vi "main 0.9.4.testing.vi"() -> ()   [LabVIEW 2020]
uses:
  subvi/Newport ESP301/Newport ESP301.lvlib
  subvi/sp_manip.llb/sp_manip_lib.lvlib
  subvi/sp_manip.llb/tcp_gateway.lvlib
  subvi/PHOIBOS/DEFINITIONS/DEF_dev_type.ctl
  subvi/PHOIBOS/DEFINITIONS/DEF_dev_state.ctl
  <vilib>/Utility/file.llb/Write Delimited Spreadsheet (DBL).vi
  <vilib>/Utility/file.llb/Read Delimited Spreadsheet (string).vi
  <vilib>/Analysis/NI_AALBase.lvlib
  <vilib>/Analysis/1siggen.llb/Ramp Pattern by Samples.vi
  <vilib>/DAQmx/create/channels.llb/DAQmx Create Channel (AI-Voltage-Basic).vi
  <vilib>/DAQmx/read.llb/DAQmx Read (Analog DBL 1Chan 1Samp).vi
panel:
  out "Pics L":i32
  out "Pics NL":i32
  out "Voltage":dbl format="%0.2f"
  out "sideimg 2":dbl[][](graph)
  in  "Frame trigger \n(High Performance and QE only)":u16
  in  "Operating mode\nHP & QE / HS & DiCam Pro":u32
  out "Waveform Chart":dbl(graph)
  out "G2 X":cluster{dbl[], "Ramp Pattern":dbl[]}(graph)={array[344 elements], "Ramp Pattern"=[5593.0, 5541.0, 5578.0, 5573.0, 5542.0, 5582.0, 5523.0, 5570.0, 5578.0, 5560.0, 5581.0, 5542.0, 5577.0, 5517.0, 5599.0, 5558.0, 5549.0, 5571.0, 5527.0, 5574.0, 5565.0, 5561.0, 5570.0, 5531.0, 5576.0, 5531.0, 5576.0, 5554.0, 5523.0, 5573.0, 5536.0, 5555.0, 5539.0, 5549.0, 5543.0, 5541.0, 5581.0, 5523.0, 5548.0, 5528.0, 5558.0, 5565.0, 5537.0, 5556.0, 5521.0, 5538.0, 5549.0, 5532.0, 5562.0, 5512.0, 5555.0, 5549.0, 5536.0, 5542.0, 5511.0, 5567.0, 5526.0, 5549.0, 5545.0, 5543.0, 5562.0, 5518.0, 5561.0, 5490.0, 5542.0, 5522.0, 5529.0, 5542.0, 5521.0, 5556.0, 5511.0, 5541.0, 5534.0, 5512.0, 5569.0, 5525.0, 5547.0, 5507.0, 5533.0, 5533.0, 5501.0, 5555.0, 5497.0, 5517.0, 5526.0, 5519.0, 5565.0, 5503.0, 5548.0, 5496.0, 5544.0, 5523.0, 5534.0, 5533.0, 5501.0, 5529.0, 5494.0, 5523.0, 5526.0, 5519.0, 5539.0, 5493.0, 5508.0, 5532.0, 5504.0, 5546.0, 5540.0, 5550.0, 5488.0, 5556.0, 5535.0, 5510.0, 5535.0, 5515.0, 5543.0, 5475.0, 5538.0, 5528.0, 5504.0, 5523.0, 5502.0, 5535.0, 5473.0, 5503.0, 5501.0, 5531.0, 5525.0, 5490.0, 5524.0, 5484.0, 5520.0, 5506.0, 5492.0, 5516.0, 5477.0, 5511.0, 5487.0, 5509.0, 5496.0, 5467.0, 5538.0, 5494.0, 5512.0, 5497.0, 5498.0, 5526.0, 5482.0, 5506.0, 5466.0, 5522.0, 5489.0, 5512.0, 5518.0, 5475.0, 5547.0, 5480.0, 5569.0, 5504.0, 5485.0, 5528.0, 5506.0, 5529.0, 5468.0, 5524.0, 5507.0, 5518.0, 5511.0, 5471.0, 5525.0, 5480.0, 5482.0, 5510.0, 5506.0, 5522.0, 5475.0, 5540.0, 5477.0, 5511.0, 5514.0, 5500.0, 5497.0, 5484.0, 5536.0, 5476.0, 5485.0, 5527.0, 5509.0, 5529.0, 5495.0, 5504.0, 5496.0, 5519.0, 5512.0, 5469.0, 5506.0, 5465.0, 5502.0, 5481.0, 5508.0, 5519.0, 5499.0, 5515.0, 5476.0, 5496.0, 5502.0, 5499.0, 5494.0, 5477.0, 5541.0, 5477.0, 5512.0, 5497.0, 5472.0, 5511.0, 5471.0, 5503.0, 5507.0, 5504.0, 5477.0, 5479.0, 5508.0, 5481.0, 5522.0, 5517.0, 5516.0, 5505.0, 5502.0, 5491.0, 5481.0, 5512.0, 5484.0, 5500.0, 5478.0, 5493.0, 5529.0, 5492.0, 5518.0, 5471.0, 5518.0, 5490.0, 5513.0, 5497.0, 5488.0, 5517.0, 5477.0, 5524.0, 5464.0, 5495.0, 5514.0, 5495.0, 5522.0, 5477.0, 5490.0, 5535.0, 5489.0, 5491.0, 5491.0, 5515.0, 5473.0, 5504.0, 5505.0, 5515.0, 5510.0, 5473.0, 5521.0, 5475.0, 5537.0, 5499.0, 5505.0, 5509.0, 5460.0, 5509.0, 5473.0, 5489.0, 5500.0, 5464.0, 5522.0, 5471.0, 5528.0, 5475.0, 5502.0, 5494.0, 5511.0, 5516.0, 5486.0, 5528.0, 5471.0, 5492.0, 5477.0, 5491.0, 5531.0, 5486.0, 5549.0, 5498.0, 5524.0, 5482.0, 5495.0, 5505.0, 5476.0, 5512.0, 5444.0, 5512.0, 5498.0, 5471.0, 5489.0, 5462.0, 5502.0, 5459.0, 5503.0, 5489.0, 5493.0, 5498.0, 5461.0, 5505.0, 5495.0, 5503.0, 5459.0, 5501.0, 5515.0, 5459.0, 5510.0, 5469.0, 5504.0, 5499.0, 5505.0, 5524.0, 5477.0, 5527.0, 5477.0, 5475.0, 5495.0, 5482.0, 5514.0, 5481.0, 5499.0, 5481.0, 5482.0, 5498.0, 5460.0, 5469.0, 5471.0, 5519.0, 5495.0, 5485.0]}
  in  "reset every n pics":bool
  in  "pics2avg":i32=50
  in  "abort acq.":bool
  out "G2 Y":cluster{dbl[], "Ramp Pattern":dbl[]}(graph)={[5738.0, 5692.0, 5562.0, 5630.0, 5633.0, 5616.0, 5523.0, 5622.0, 5406.0, 5598.0, 5416.0, 5403.0, 5579.0, 5325.0, 5504.0, 5402.0, 5538.0, 5568.0, 5460.0, 5494.0, 5367.0, 5597.0, 5434.0, 5448.0, 5339.0, 5434.0, 5460.0, 5482.0, 5646.0, 5720.0, 5704.0, 5628.0, 5672.0, 5511.0, 5420.0, 5539.0, 5543.0, 5421.0, 5486.0, 5508.0, 5537.0, 5586.0, 5460.0, 5547.0, 5433.0, 5488.0, 5552.0, 5538.0, 5528.0, 5482.0, 5406.0, 5458.0, 5644.0, 5485.0, 5443.0, 5485.0, 5385.0, 5413.0, 5472.0, 5571.0, 5640.0, 5602.0, 5462.0, 5477.0, 5408.0, 5396.0, 5445.0, 5638.0, 5383.0, 5571.0, 5372.0, 5519.0, 5426.0, 5462.0, 5481.0, 5626.0, 5326.0, 5458.0, 5471.0, 5366.0, 5394.0, 5363.0, 5551.0, 5596.0, 5452.0, 5470.0, 5600.0, 5533.0, 5573.0, 5544.0, 5671.0, 5595.0, 5423.0, 5550.0, 5557.0, 5416.0, 5404.0, 5478.0, 5448.0, 5512.0, 5505.0, 5575.0, 5434.0, 5436.0, 5600.0, 5487.0, 5607.0, 5463.0, 5606.0, 5540.0, 5521.0, 5581.0, 5472.0, 5555.0, 5576.0, 5612.0, 5529.0, 5473.0, 5454.0, 5455.0, 5500.0, 5650.0, 5451.0, 5445.0, 5423.0, 5376.0, 5389.0, 5491.0, 5536.0, 5525.0, 5440.0, 5707.0, 5414.0, 5532.0, 5400.0, 5668.0, 5706.0, 5515.0, 5431.0, 5400.0, 5439.0, 5471.0, 5627.0, 5691.0, 5569.0, 5718.0, 5614.0, 5523.0, 5436.0, 5432.0, 5419.0, 5516.0, 5469.0, 5467.0, 5530.0, 5598.0, 5501.0, 5476.0, 5457.0, 5460.0, 5606.0, 5456.0, 5429.0, 5586.0, 5504.0, 5546.0, 5516.0, 5466.0, 5650.0, 5593.0, 5605.0, 5515.0, 5414.0, 5623.0, 5581.0, 5651.0, 5574.0, 5519.0, 5672.0, 5621.0, 5496.0, 5382.0, 5496.0, 5620.0, 5542.0, 5422.0, 5492.0, 5515.0, 5549.0, 5402.0, 5472.0, 5547.0, 5515.0, 5641.0, 5451.0, 5667.0, 5622.0, 5511.0, 5506.0, 5608.0, 5647.0, 5584.0, 5714.0, 5490.0, 5534.0, 5463.0, 5566.0, 5573.0, 5570.0, 5582.0, 5613.0, 5504.0, 5550.0, 5594.0, 5576.0, 5677.0, 5675.0, 5681.0, 5681.0, 5434.0, 5434.0, 5405.0, 5473.0, 5522.0, 5427.0, 5533.0, 5582.0, 5427.0, 5529.0, 5548.0, 5341.0, 5521.0, 5539.0, 5435.0, 5457.0, 5511.0, 5406.0, 5412.0, 5620.0, 5609.0, 5609.0, 5469.0, 5577.0, 5661.0, 5673.0, 5518.0, 5463.0, 5562.0, 5723.0, 5719.0, 5487.0, 5485.0, 5683.0, 5501.0, 5604.0, 5328.0], "Ramp Pattern"=[0.0, 1.003921568627451, 2.007843137254902, 3.011764705882353, 4.015686274509804, 5.019607843137255, 6.023529411764706, 7.027450980392157, 8.031372549019608, 9.035294117647059, 10.03921568627451, 11.04313725490196, 12.047058823529412, 13.050980392156863, 14.054901960784314, 15.058823529411764, 16.062745098039215, 17.066666666666666, 18.070588235294117, 19.07450980392157, 20.07843137254902, 21.08235294117647, 22.08627450980392, 23.090196078431372, 24.094117647058823, 25.098039215686274, 26.101960784313725, 27.105882352941176, 28.109803921568627, 29.113725490196078, 30.11764705882353, 31.12156862745098, 32.12549019607843, 33.129411764705885, 34.13333333333333, 35.13725490196079, 36.141176470588235, 37.14509803921569, 38.14901960784314, 39.15294117647059, 40.15686274509804, 41.16078431372549, 42.16470588235294, 43.168627450980395, 44.17254901960784, 45.1764705882353, 46.180392156862744, 47.1843137254902, 48.188235294117646, 49.1921568627451, 50.19607843137255, 51.2, 52.20392156862745, 53.207843137254905, 54.21176470588235, 55.21568627450981, 56.219607843137254, 57.22352941176471, 58.227450980392156, 59.23137254901961, 60.23529411764706, 61.23921568627451, 62.24313725490196, 63.247058823529414, 64.25098039215686, 65.25490196078431, 66.25882352941177, 67.26274509803922, 68.26666666666667, 69.27058823529411, 70.27450980392157, 71.27843137254902, 72.28235294117647, 73.28627450980392, 74.29019607843138, 75.29411764705883, 76.29803921568627, 77.30196078431372, 78.30588235294118, 79.30980392156863, 80.31372549019608, 81.31764705882352, 82.32156862745099, 83.32549019607843, 84.32941176470588, 85.33333333333333, 86.33725490196079, 87.34117647058824, 88.34509803921569, 89.34901960784313, 90.3529411764706, 91.35686274509804, 92.36078431372549, 93.36470588235294, 94.3686274509804, 95.37254901960785, 96.37647058823529, 97.38039215686274, 98.3843137254902, 99.38823529411765, 100.3921568627451, 101.39607843137254, 102.4, 103.40392156862745, 104.4078431372549, 105.41176470588235, 106.41568627450981, 107.41960784313726, 108.4235294117647, 109.42745098039215, 110.43137254901961, 111.43529411764706, 112.43921568627451, 113.44313725490196, 114.44705882352942, 115.45098039215686, 116.45490196078431, 117.45882352941176, 118.46274509803922, 119.46666666666667, 120.47058823529412, 121.47450980392156, 122.47843137254903, 123.48235294117647, 124.48627450980392, 125.49019607843137, 126.49411764705883, 127.49803921568628, 128.50196078431372, 129.50588235294117, 130.50980392156862, 131.51372549019607, 132.51764705882354, 133.521568627451, 134.52549019607844, 135.52941176470588, 136.53333333333333, 137.53725490196078, 138.54117647058823, 139.54509803921567, 140.54901960784315, 141.5529411764706, 142.55686274509804, 143.5607843137255, 144.56470588235294, 145.5686274509804, 146.57254901960783, 147.57647058823528, 148.58039215686276, 149.5843137254902, 150.58823529411765, 151.5921568627451, 152.59607843137255, 153.6, 154.60392156862744, 155.6078431372549, 156.61176470588236, 157.6156862745098, 158.61960784313726, 159.6235294117647, 160.62745098039215, 161.6313725490196, 162.63529411764705, 163.6392156862745, 164.64313725490197, 165.64705882352942, 166.65098039215687, 167.65490196078431, 168.65882352941176, 169.6627450980392, 170.66666666666666, 171.6705882352941, 172.67450980392158, 173.67843137254903, 174.68235294117648, 175.68627450980392, 176.69019607843137, 177.69411764705882, 178.69803921568626, 179.7019607843137, 180.7058823529412, 181.70980392156864, 182.71372549019608, 183.71764705882353, 184.72156862745098, 185.72549019607843, 186.72941176470587, 187.73333333333332, 188.7372549019608, 189.74117647058824, 190.7450980392157, 191.74901960784314, 192.75294117647059, 193.75686274509803, 194.76078431372548, 195.76470588235293, 196.7686274509804, 197.77254901960785, 198.7764705882353, 199.78039215686275, 200.7843137254902, 201.78823529411764, 202.7921568627451, 203.79607843137254, 204.8, 205.80392156862746, 206.8078431372549, 207.81176470588235, 208.8156862745098, 209.81960784313725, 210.8235294117647, 211.82745098039214, 212.83137254901962, 213.83529411764707, 214.8392156862745, 215.84313725490196, 216.8470588235294, 217.85098039215686, 218.8549019607843, 219.85882352941175, 220.86274509803923, 221.86666666666667, 222.87058823529412, 223.87450980392157, 224.87843137254902, 225.88235294117646, 226.8862745098039, 227.89019607843136, 228.89411764705883, 229.89803921568628, 230.90196078431373, 231.90588235294118, 232.90980392156862, 233.91372549019607, 234.91764705882352, 235.92156862745097, 236.92549019607844, 237.9294117647059, 238.93333333333334, 239.93725490196078, 240.94117647058823, 241.94509803921568, 242.94901960784313, 243.95294117647057, 244.95686274509805, 245.9607843137255, 246.96470588235294, 247.9686274509804, 248.97254901960784, 249.9764705882353, 250.98039215686273, 251.98431372549018, 252.98823529411766, 253.9921568627451, 254.99607843137255, 256.0]}
  out "ETA":timestamp=timestamp(3543843884.995538 s since 1904-01-01) format="%<%H:%M:%S>T"
  out "acq. imgs":i32=30
  out "snap_prog":dbl(slide)=1.0 scale=0.0..1.0
  in  "BasePath":path=path "Z:/PESdata"
  in  "cam_liveavg":bool caption="live average"
  out "cam_fps":dbl=20.079713544692744 caption="FPS" format="%.1g"
  out "sideimg":dbl[][](graph)
  in  "RunNumber":u16=77
  out "sum":dbl=4126991.0 format="%#.2g"
  out "max":dbl=54.0
  out "mainimg":dbl[][](graph)
  out "ESP_con?":bool=TRUE caption="ESP301"
  out "phoib_con?":bool caption="PHOIBOS"
  out "manip_con?":bool caption="manipulator"
  out "cam_con?":bool caption="camera"
  in  "main_close":bool
  in  "Tab Control":T1(tab)
  in  "manip_deltas":dbl[](array[numeric])=[0.0, 0.0, 0.0, 0.0, 10.0, 0.0] caption="delta" format="%#.5g"
  in  "aq.mode":enum32{"Radio Selection 1", "Radio Selection 2"}(radio)=enum."Radio Selection 2"
  in  "dark avg":i32=100
  in  "averages":i32=30 caption="N"
  in  "ESP_delta":dbl caption="relative [mm]"
  in  "ESP_-":bool
  in  "ESP_+":bool
  in  "ESP_go":bool
  in  "ESP_dest_t":dbl=250.17307139859977 caption="[fs]"
  in  "ESP_dest":dbl=31.304 caption="[mm]"
  in  "ESP_set_t0":bool
  in  "phoib_I_6s":dbl=3200.0
  in  "phoib_I_5s":dbl=1650.0
  in  "phoib_I_4s":dbl=4.558
  in  "phoib_I_3s":dbl=-7.0
  in  "phoib_I_2s":dbl=20.0
  in  "phoib_I_1s":dbl=22.0
  in  "phoib_standby":bool
  in  "phoib_set":bool
  out "phoib_I_6":dbl caption="Screen Voltage"
  out "phoib_I_5":dbl caption="Detctor Voltage"
  out "phoib_I_4":dbl caption="Work Function"
  out "phoib_I_3":dbl caption="Coil Current"
  out "phoib_I_2":dbl caption="Pass Energy"
  out "phoib_I_1":dbl caption="Kinetic Energy"
  out "Saved Positions":string[][](table)=[["ertwertwert", "-2.299945", "-2.030214", "38.900024", "50.000762", "0.000887", "-97.998082"], ["uztgugt", "-14.999451", "-13.638894", "442.380066", "13.998380", "-1.893758", "-76.305838"], ["asdf", "-14.999451", "-13.638894", "442.380066", "13.998380", "-1.893758", "-76.305838"], ["test3", "-14.999451", "-13.638894", "441.380066", "13.998380", "-1.893758", "-76.305838"]]
  in  "Save Pos":bool
  in  "Load":bool
  in  "Delete":bool
  in  "ManipRel +":bool
  in  "ManipRel -":bool
  in  "Move Abs":bool
  in  "stop manip":bool
  in  "dest":dbl[](array[numeric])=[-2.6172862113166087, -0.009888298846365134, 68.5008544921875, -46.36280498847848, 1.1073518432055398, -218.56360350415366] caption="destination" format="%#.5g"
  out "axis":string[](array[string])=["x", "y", "z", "polar", "tilt", "azimut"]
  out "pos":dbl[](array[numeric])=[-2.6172862113166087, -0.009888298846365134, 68.5008544921875, -46.363686276590336, 11.108982061941884, -218.56360350415366] caption="position" format="%.5f"
  in  "Mode":T2(ring)=enum."WideAngleMode"
  in  "VoltageRange":enum16{"3.5kV", "1.5kV", "400V", "100V", "10V"}(ring)=enum."400V"
  out "ESP_pos":dbl=31.4539 caption="Position"
  out "ESP_delay":dbl=1000.0251574040756 caption="Delay"
  out "ESP_t0":dbl=31.304 caption="Time Zero @"
  out "phoib_I_7":dbl caption="Conversion Voltage"
  in  "phoib_I_7s":dbl=-16.0
  in  "phoib_I_8s":dbl=0.0039
  in  "phoib_I_9s":dbl=0.0039
  out "phoib_I_8":dbl caption="FD1"
  out "phoib_I_9":dbl caption="FD2"
  in  "gain":bool
  in  "exposure [ms]":u32=1
  in  "binning":u16(ring)=2 items=["X 1", "X 2", "X 4", "X 8"]
  in  "cam_dark?":bool caption="subtract dark?"
  in  "cam_dark":bool
  in  "cam_saveimg":bool
  in  "e-size":u8
  in  "lower threshold":i32=-100
  in  "count?":bool
  in  "ROI Left":i32=1
  in  "ROI Right":i32=43
  in  "ROI Top":i32=1
  in  "ROI Bottom":i32=33
  out "moving?":bool[](array[boolean])
  in  "delscan_abort 2":bool
  in  "delscan_go 2":bool
  in  "delscan_finishIteration 2":bool
  out "del_ETA":timestamp=timestamp(3543843871.185777 s since 1904-01-01) format="%<%H:%M:%S>T"
  out "time / step":dbl=2.792118032773336
  out "duration [HH:MM:SS]":dbl=55.62603882380894 format="%<%H:%M:%S>t"
  out "disk [MB]":dbl=11.613000000000001
  out "RAM [MB]":dbl=2.765
  out "total steps":dbl=20.0
  out "delaypoints":dbl=5.0
  in  "generate delay table":bool
  in  "load delay table":bool
  in  "delay table [fs]":string[][](table)=[["-1000.000000"], ["-500.000000"], ["0.000000"], ["500.000000"], ["1000.000000"]]
  in  "delscan_iters":u32=4 caption="iterations"
  out "scangraph":cluster{"delaypoints":dbl[], dbl[]}(graph)={"delaypoints"=[-1000.0, -500.0, 0.0, 500.0, 1000.0], [56872639.0, 56944859.59999999, 56835838.7999999, 56879783.599999934, 56864774.39999998]}
  in  "delscan_abort":bool
  out "delscan_progress":u32(slide)=5 scale=0.0..5.0
  in  "delscan_go":bool
  out "delscan_pos":dbl=31.453896228999998 caption="stage pos [mm]"
  in  "delscan_end":dbl=1000.0 caption="end [fs]"
  in  "delscan_stepsize":dbl=500.0 caption="stepsize [fs]"
  in  "delscan_start":dbl=-1000.0 caption="start [fs]"
  out "iteration":i32=5
  in  "delscan_finishIteration":bool
  in  "manip_scan_steps":u32=3
  in  "Optimize":bool
  in  "manip_scan_delta":dbl[](array[numeric])=[0.0, 0.0, 0.0, 0.0, 1.0, 0.0] caption="delta" format="%#.5g"
  out "delscan_progress 2":u32(slide)=2 scale=0.0..3.0
  in  "abort":bool
  in  "dev_bench":bool
  out "x/y":dbl
  out "1/x":dbl
  in  "stop":bool
  out "voltage out":dbl
  in  "manip_init":bool
  in  "manip_release":bool
  in  "phoib_init":bool
  in  "phoib_release":bool
  in  "ESP_init":bool
  in  "ESP_release":bool
  in  "ESP301 VISA":refnum<visa-resource-name>="COM8"
  in  "board number":i32
  in  "cam_init":bool
  in  "cam_release":bool
  out "cam_error":errorcluster
  out "phoib_error":errorcluster
  out "state":T3 items=["Off"=-1, "Standby"=0, "On"=1]
  in  "ESP Axis":i32=1 min=1 max=3
  out "error out":errorcluster
  out "error out 2":errorcluster={"status"=TRUE, "code"=1, "source"="TCP Write in sp_manip_lib.lvlib:sp_manip_disconnect.vi->main 0.9.1.vi"}
  # "0 = sequential\n1 = simultaneous"
  # "0 = internal\n1 = external rising\n2 = external falling"
  # "camera"
  # "analyzer"
  # "manipulator"
  # "aquisition"
  # "delay stage"
  # "Position"
  # "Destination"
  # "X\nY\nZ\npolar\ntilt\nazimut"
  # "camera"
  # "phoibos"
  # "ESP301"
  # "manipulator"
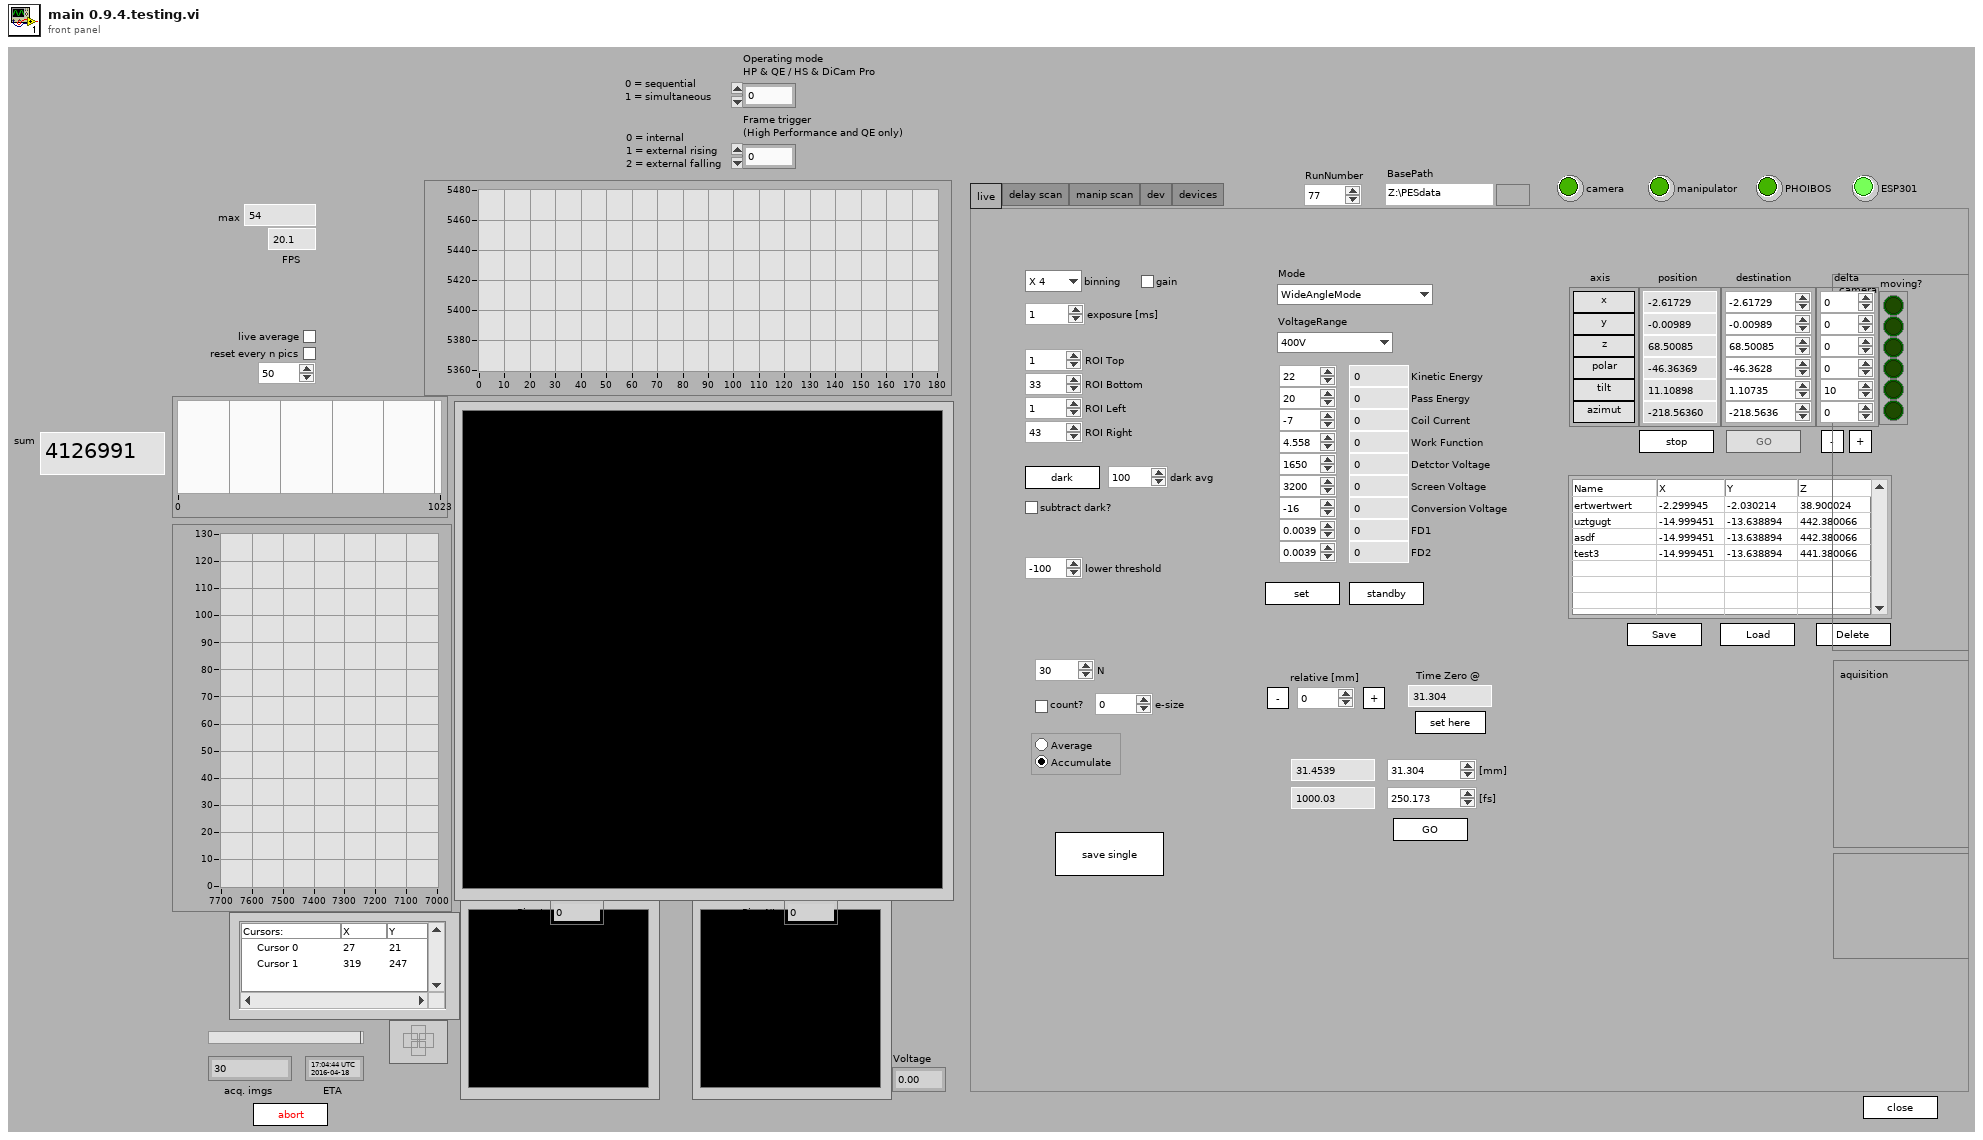
[diagram p1: front panel]
types:
  T1 = enum32{"live", "delay scan", "manip scan", "dev", "devices"}
  T2 = enum16{"HighMagnification", "MediumMagnification", "LowMagnification", "HighAngularDispersion", "MediumAngularDispersion", "LowAngularDispersion", "WideAngleMode", "LargeArea", "MediumArea", "SmallArea", "HighMagnification2", "SmallArea2", "ImagingMode"}
  T3 = typedef "DEF_dev_state.ctl" = i32
  T4 = typedef "LVCursorListTypeDef.ctl" = cluster{"Name":string, "Color":u32, "Style":u8, "Point Style":u8, "Name Visible":bool, "Allow Drag":bool, "Cursor Mode":u32, "Plot":i32, "Index":i32, "Position":cluster{"X":dbl, "Y":dbl}, "X Scale":u32, "Y Scale":u32, "Watch Plots":i32[], "Watch All Plots":bool, "Plot Area":i32, "Label Offset":cluster{"X":dbl, "Y":dbl}}[]
  T5 = cluster{"delay pointss [fs]":dbl[], "Intensity Chart":dbl[]}
  T6 = cluster{"Camera type":u32, "Operating mode\nHP & QE / HS & DiCam Pro ":u32, "Frame trigger \n(High Performance and QE only)":u16, "Sequence trigger":u16, "Low Light\n(QE only)":bool, "Gain":bool, "Horzontal\nbinning":u16, "Vertical\nbinning ":u16, "ROI Left":i32, "ROI Right":i32, "ROI Top":i32, "ROI Bottom":i32}
  T7 = cluster{"Name":string, "Color":u32, "Style":u8, "Point Style":u8, "Name Visible":bool, "Allow Drag":bool, "Cursor Mode":u32, "Plot":i32, "Index":i32, "Position":cluster{"X":dbl, "Y":dbl}, "X Scale":u32, "Y Scale":u32, "Watch Plots":i32[], "Watch All Plots":bool, "Plot Area":i32, "Label Offset":cluster{"X":dbl, "Y":dbl}}
  T8 = cluster{"Axis_Name":string, "Axis_Type":string, "Axis_Position":dbl, "continous":bool, "moving":bool}[]
  T9 = typedef "DEF_dev_type.ctl" = enum32{"devA (analyzer)", "devD (detector)"}
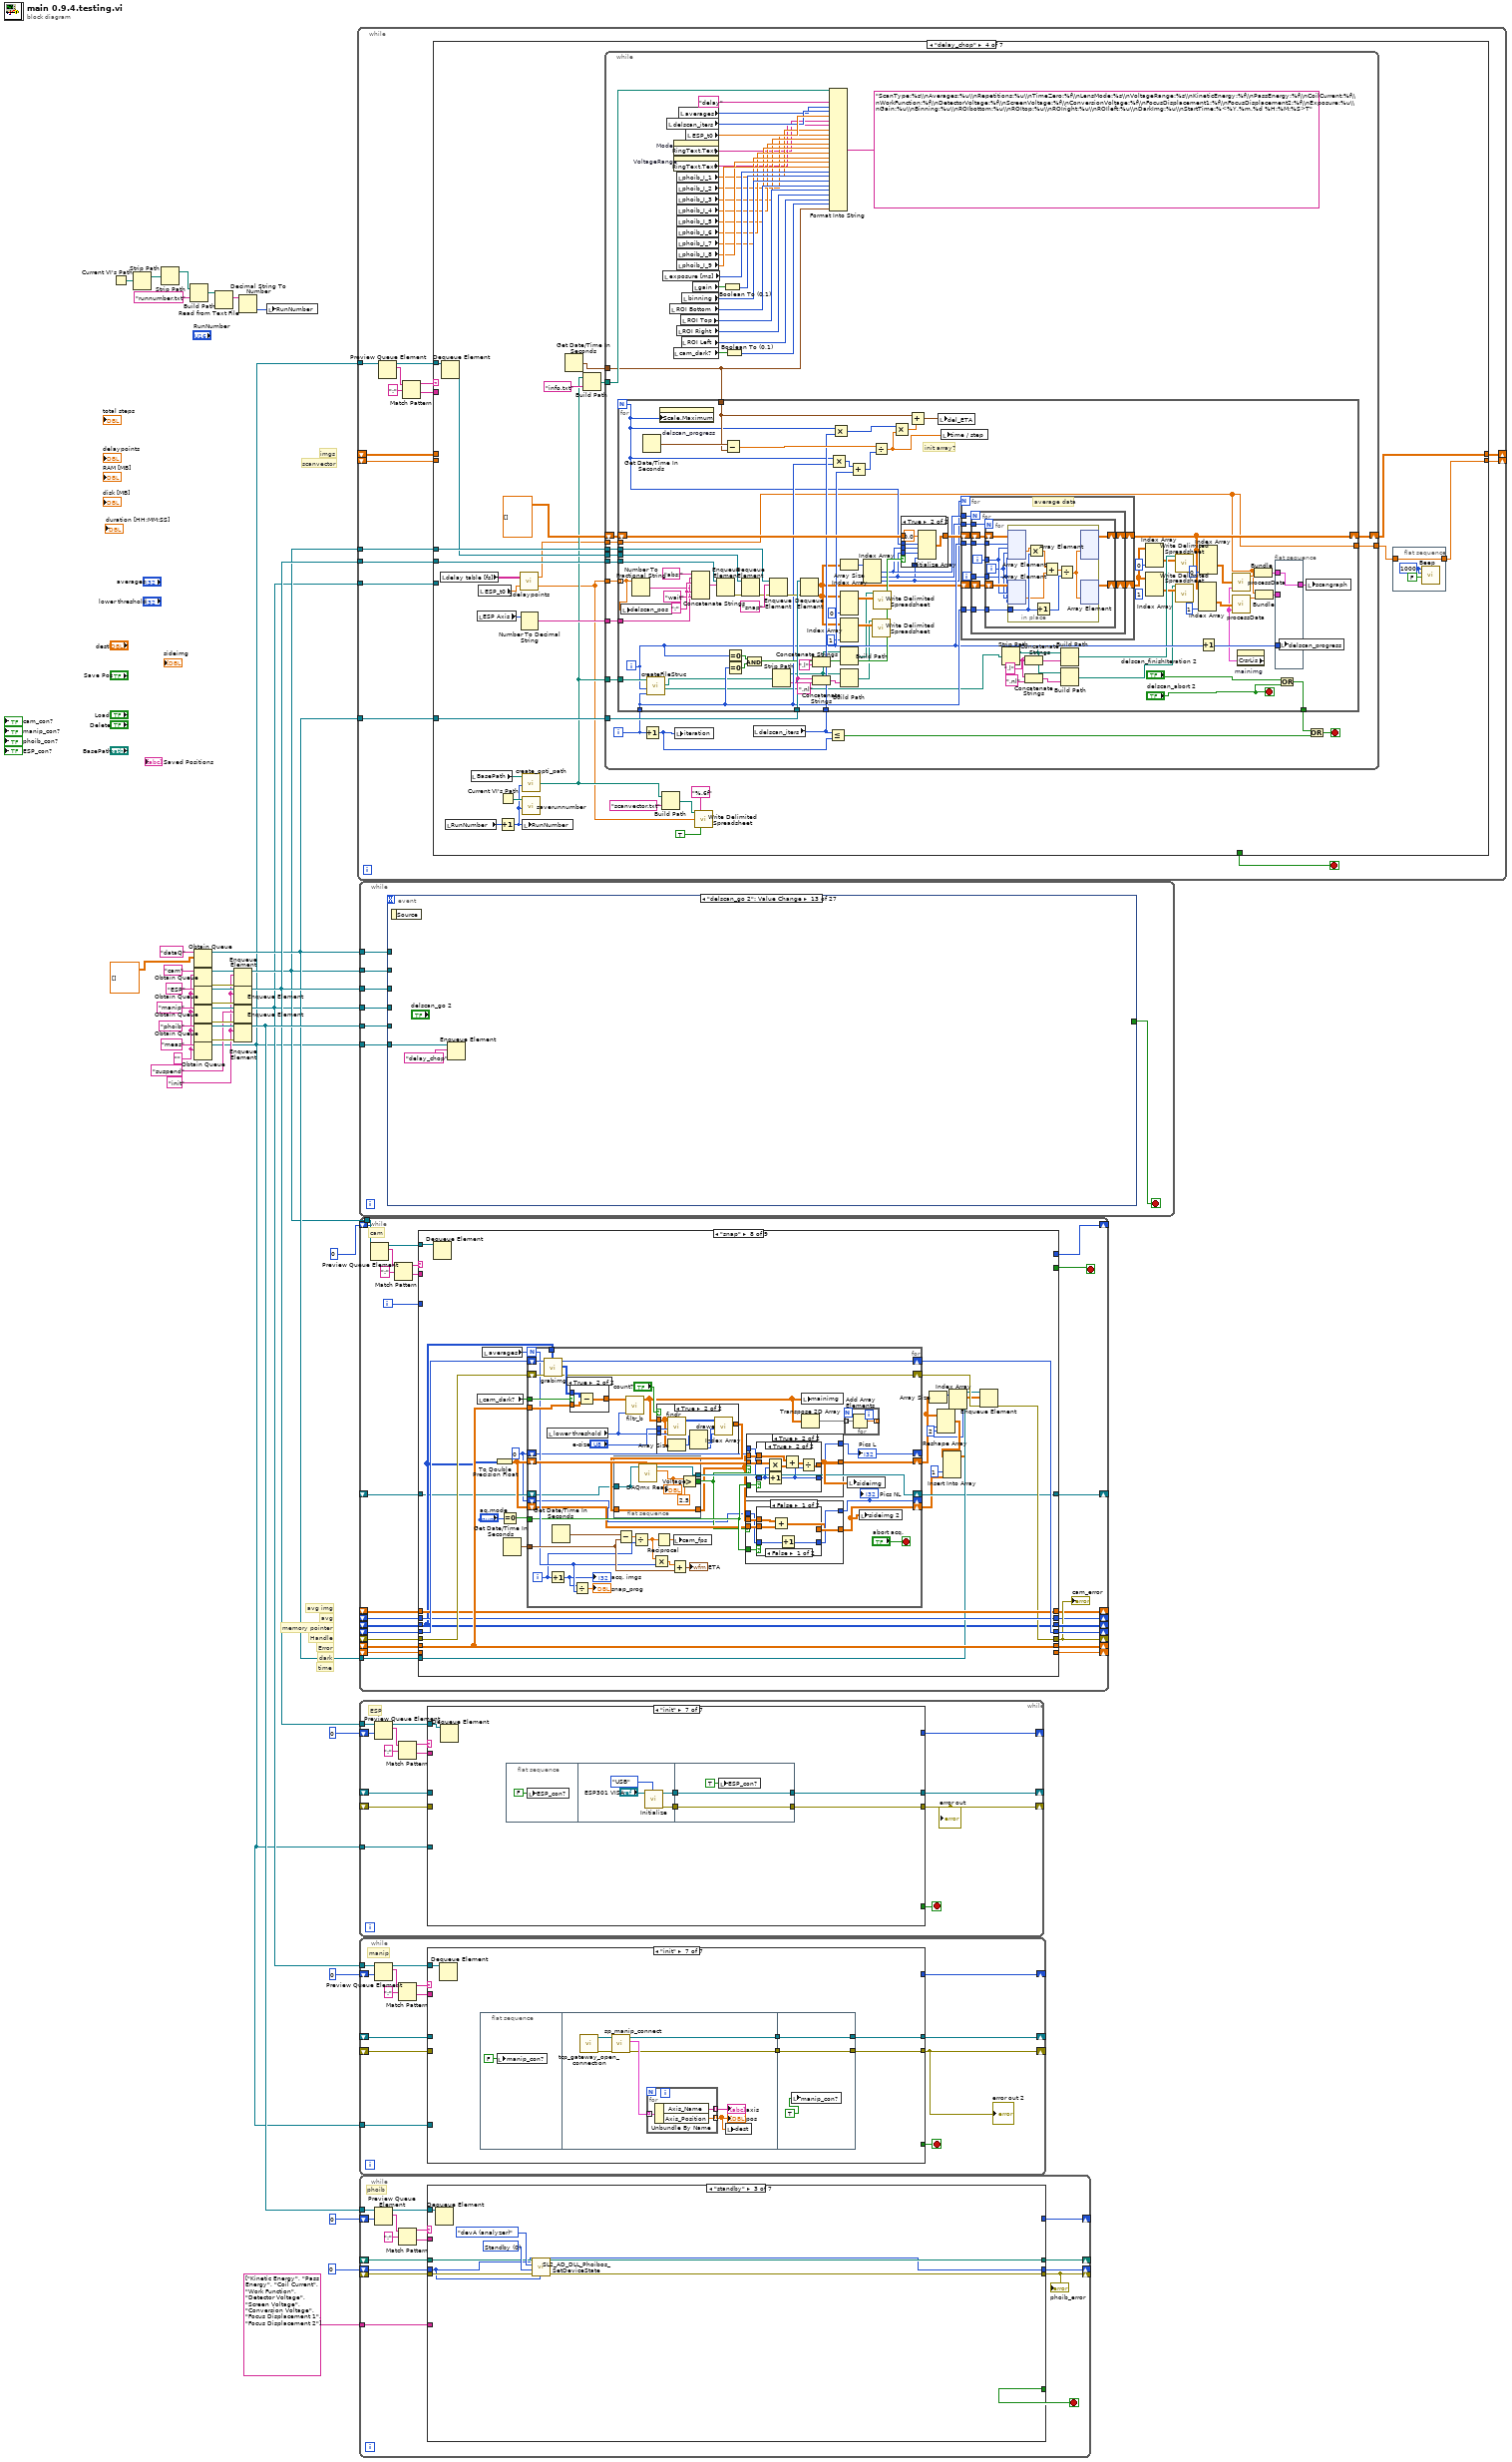
[diagram p0: block diagram]
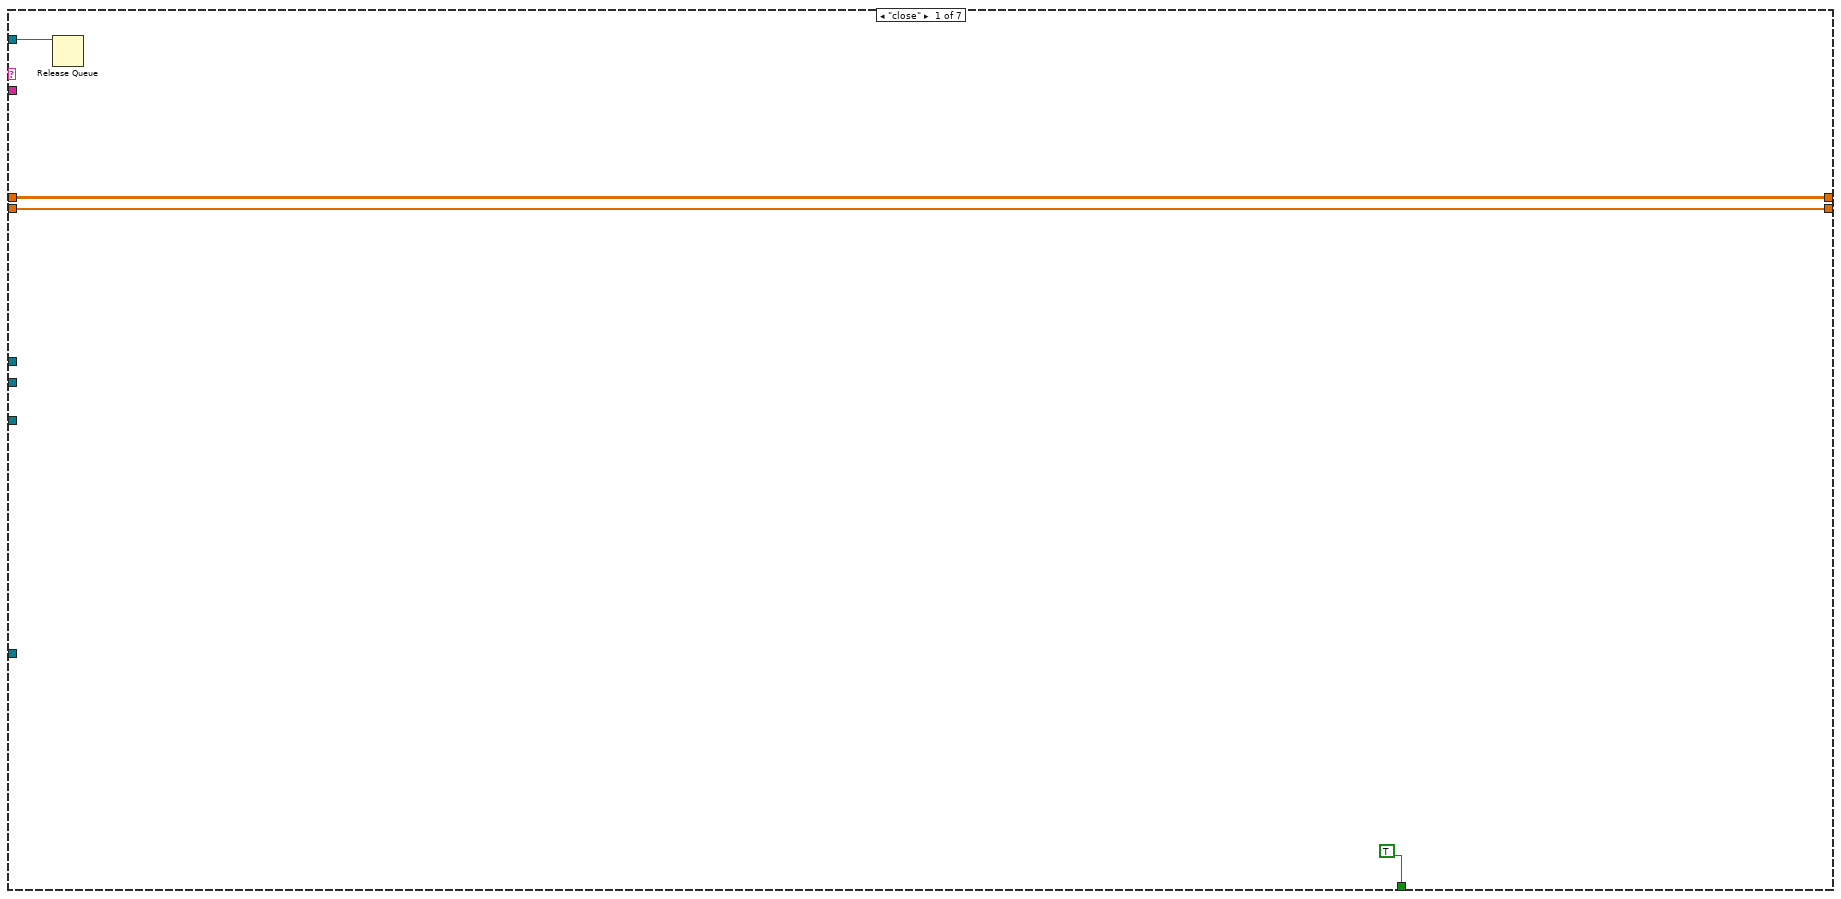
[diagram p2: hidden frame]
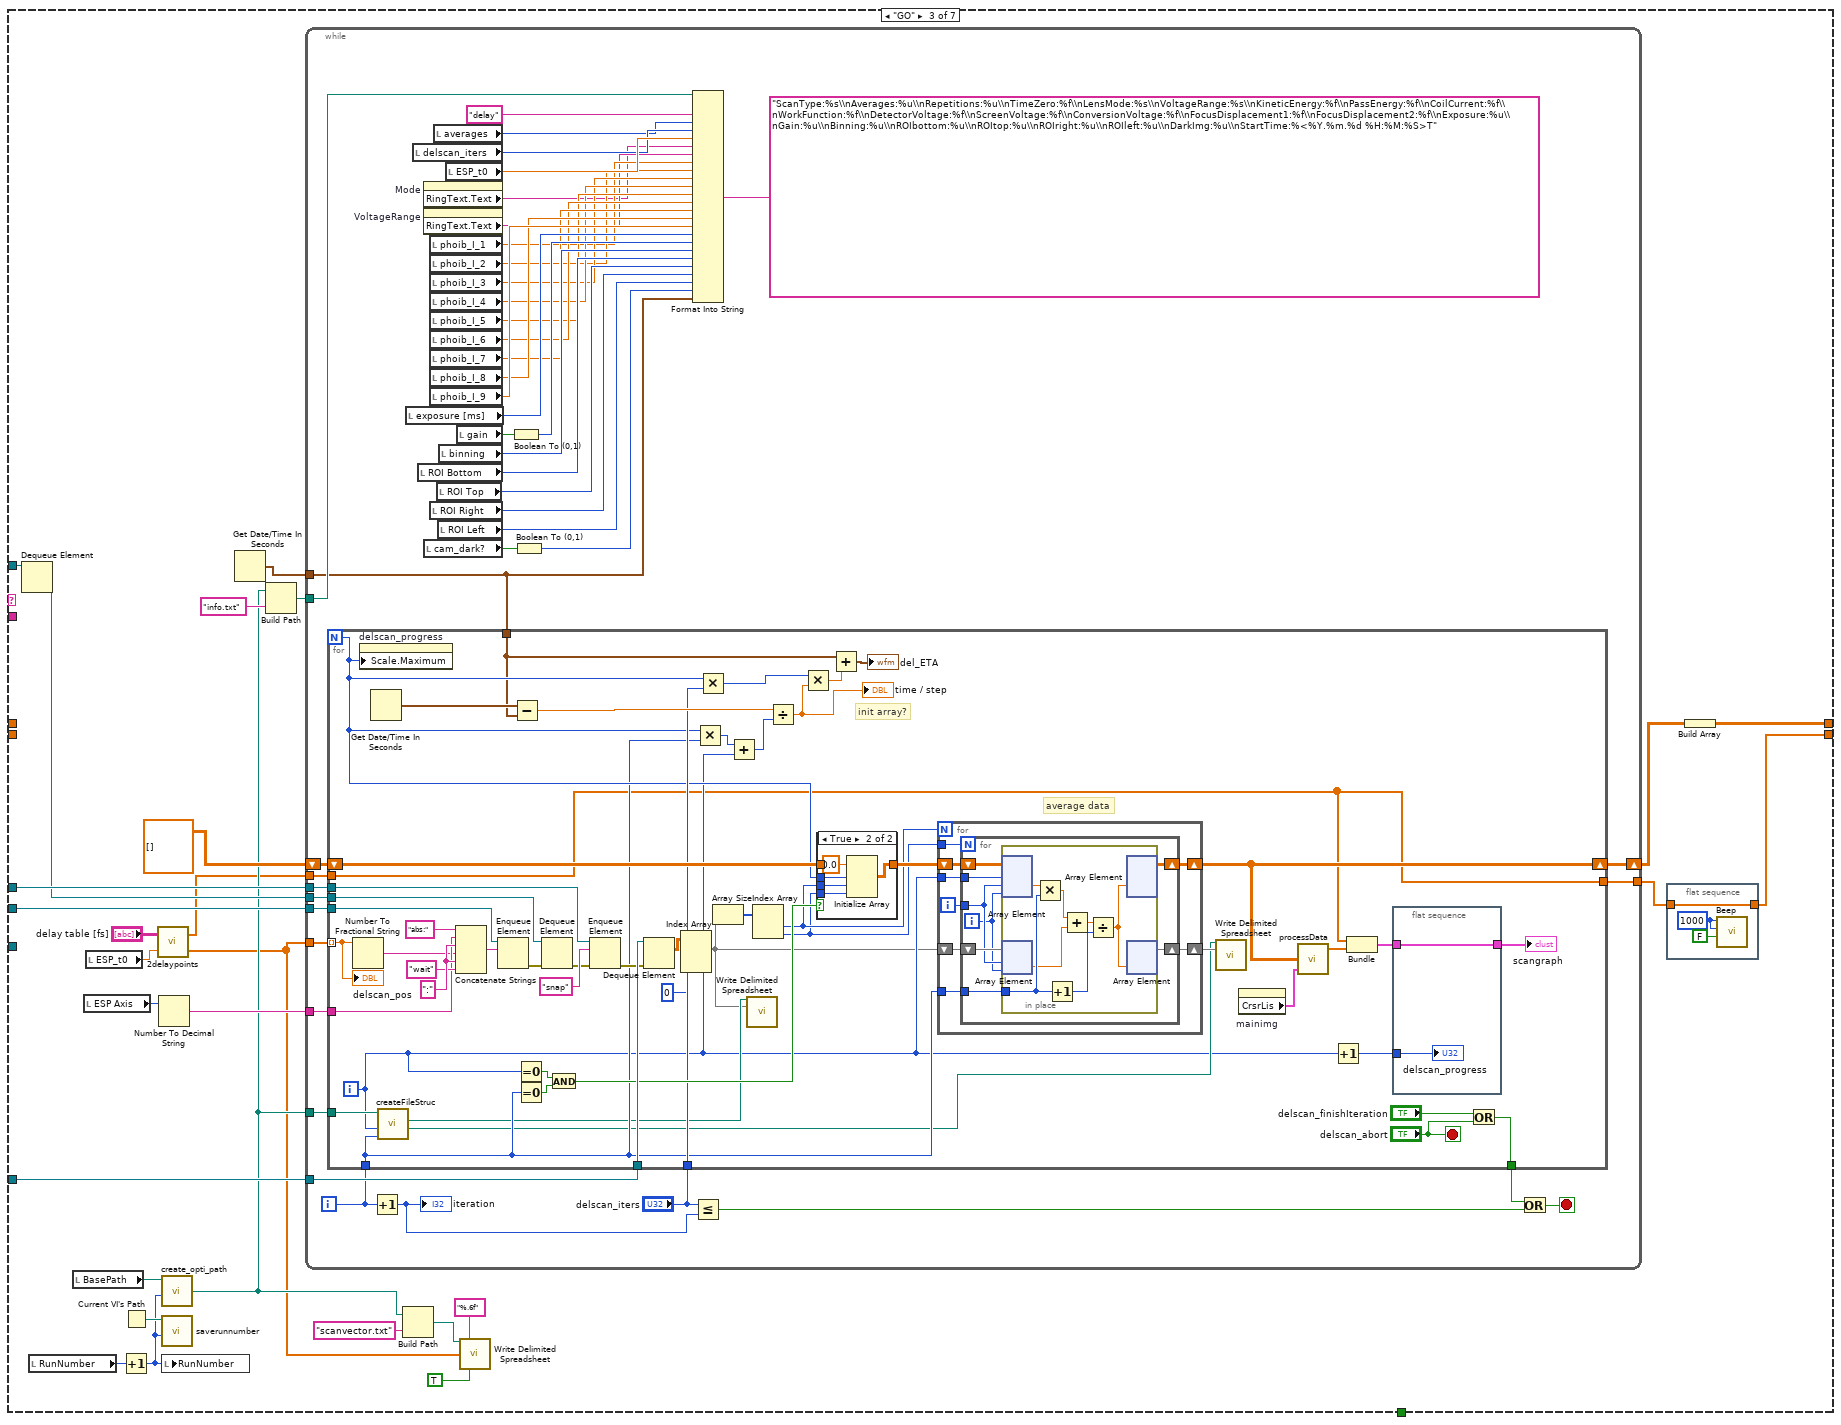
[diagram p4: hidden frame]
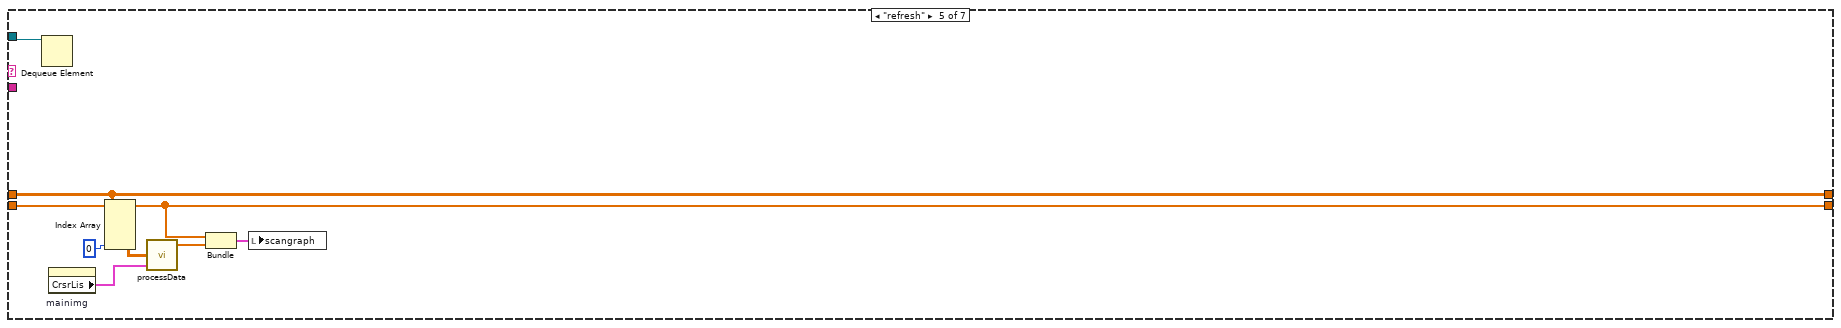
[diagram p7: hidden frame]
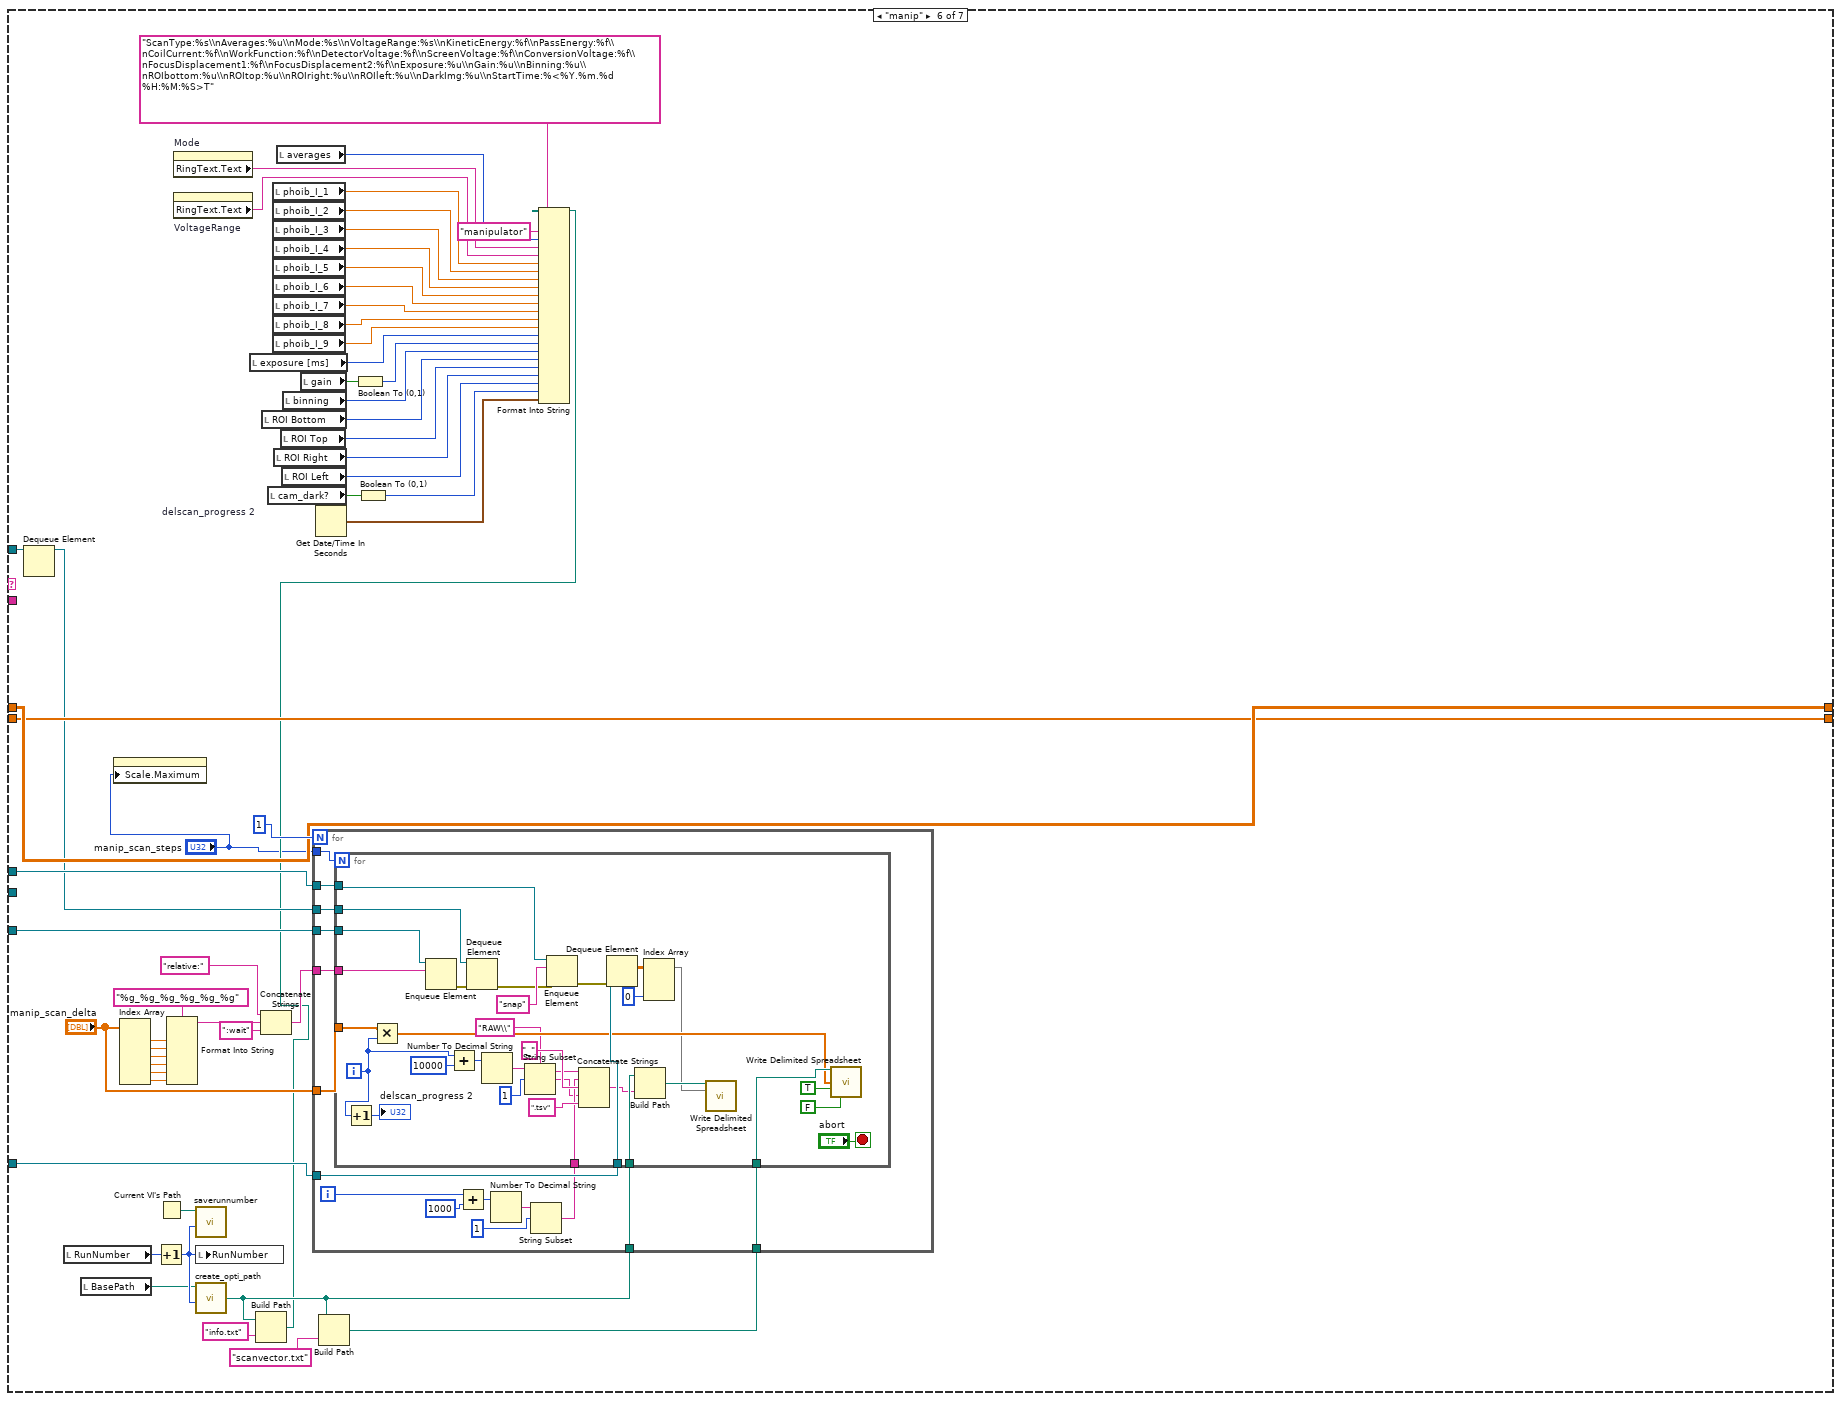
[diagram p8: hidden frame]
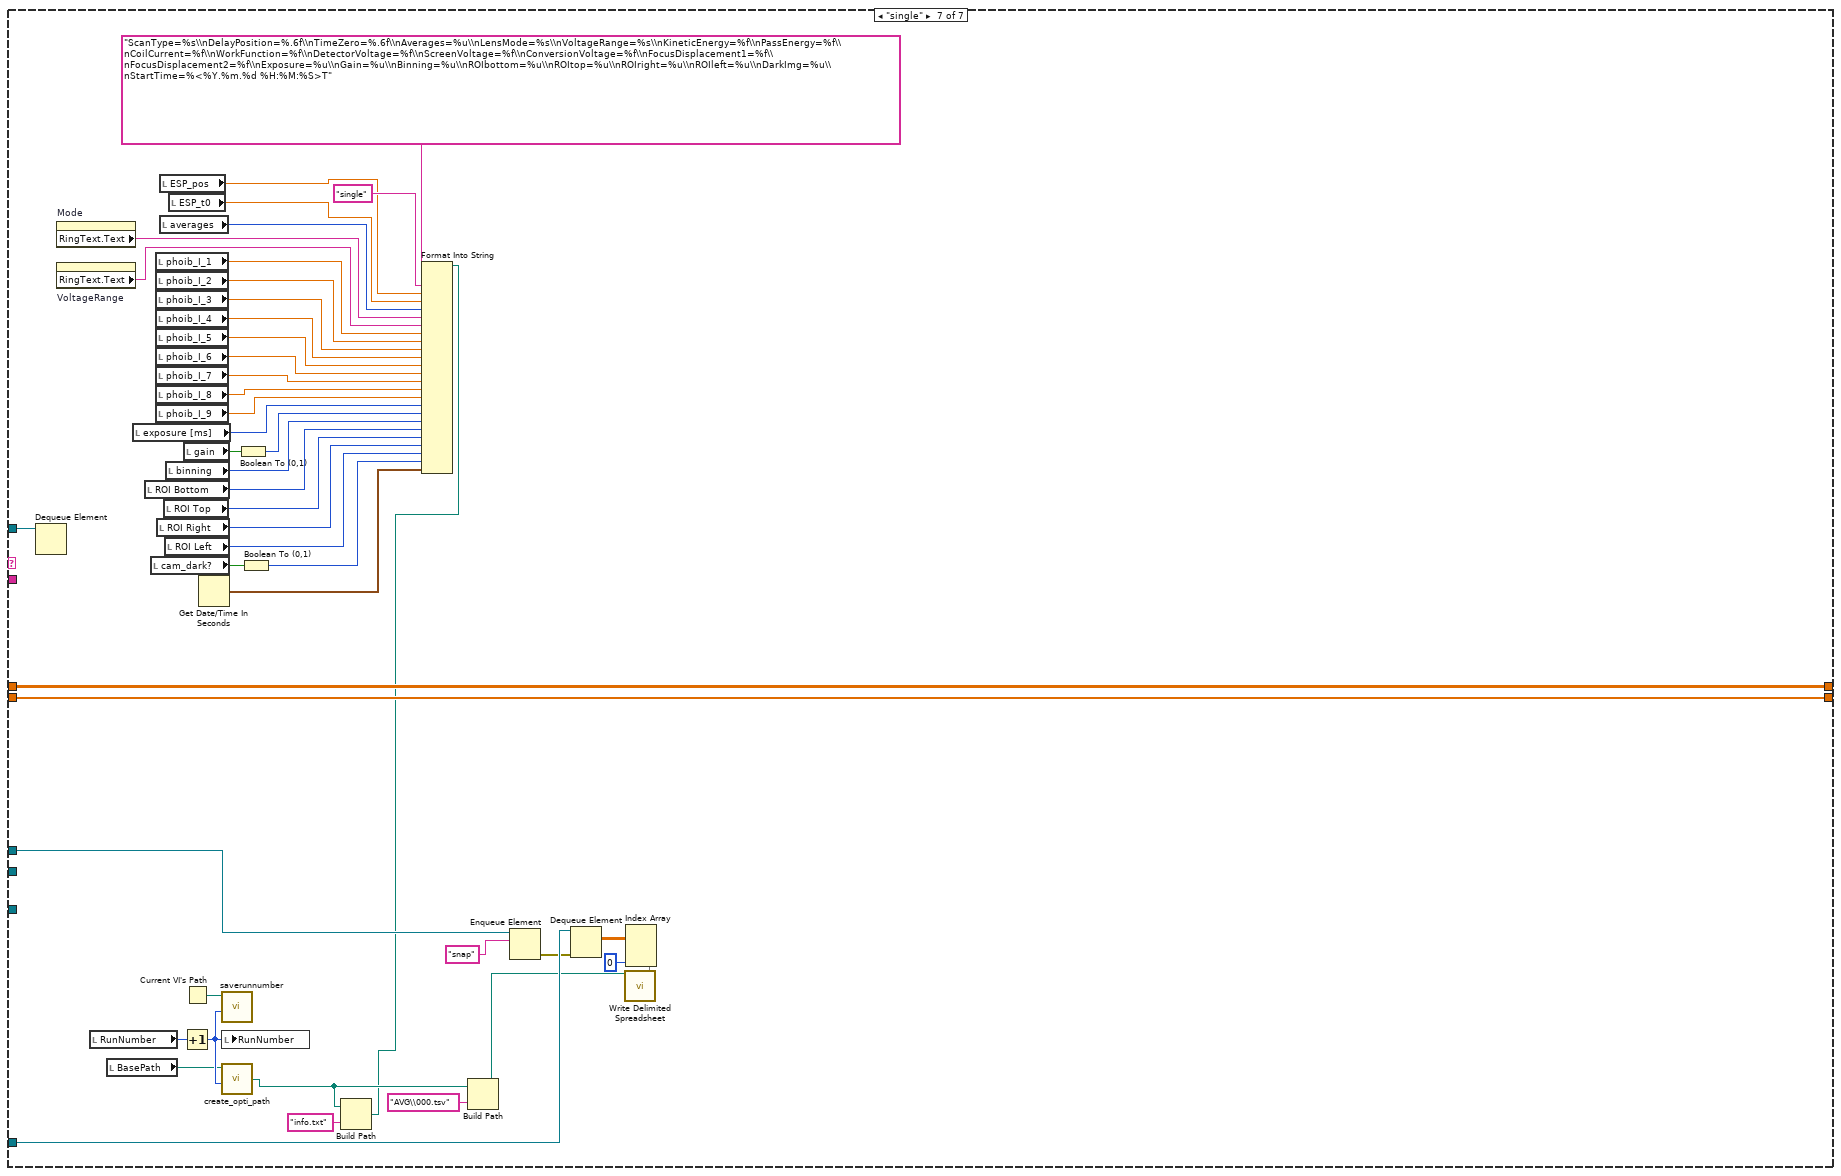
[diagram p9: hidden frame]
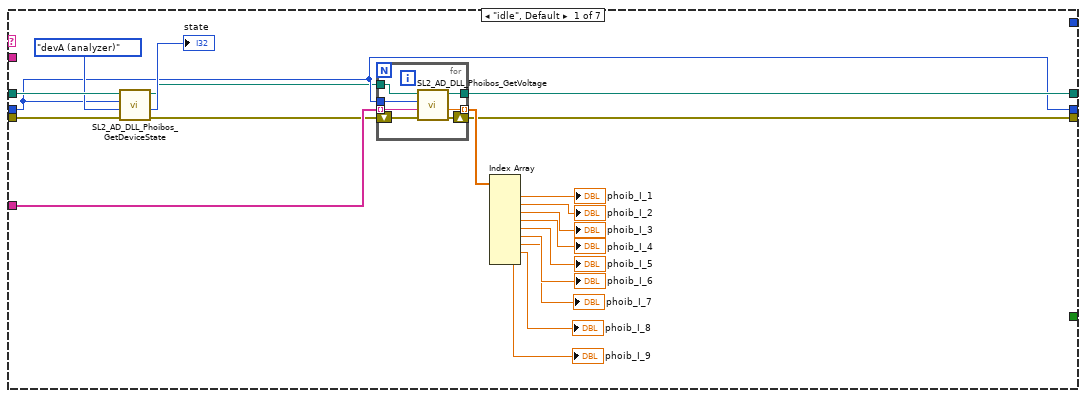
[diagram p10: hidden frame]
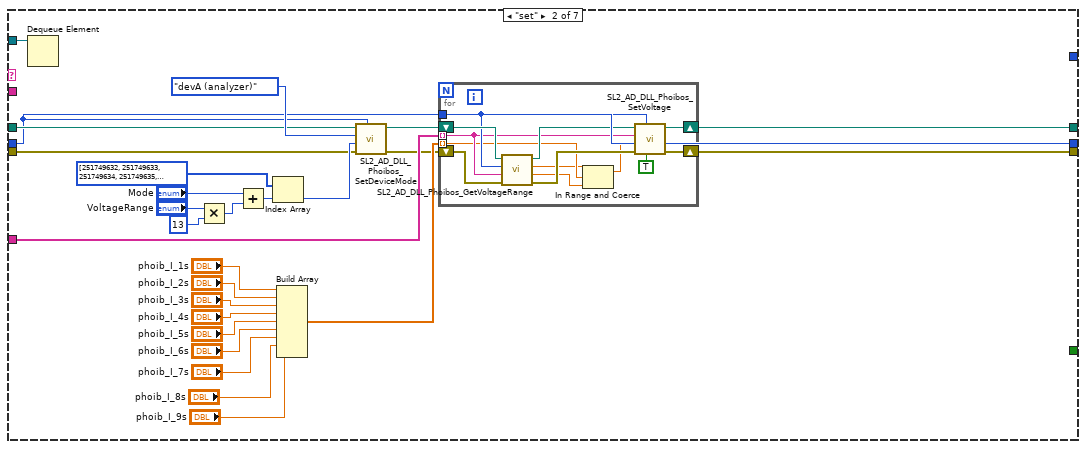
[diagram p11: hidden frame]
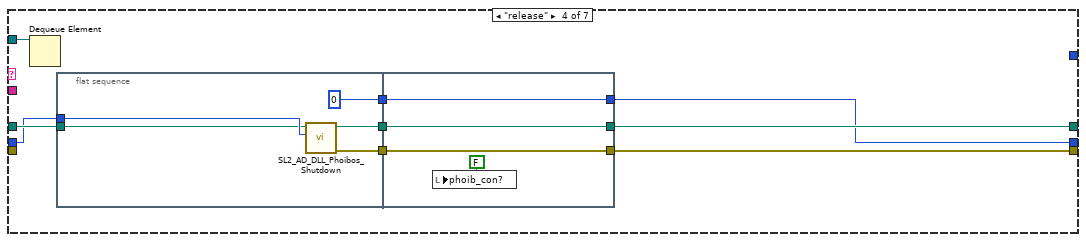
[diagram p12: hidden frame]
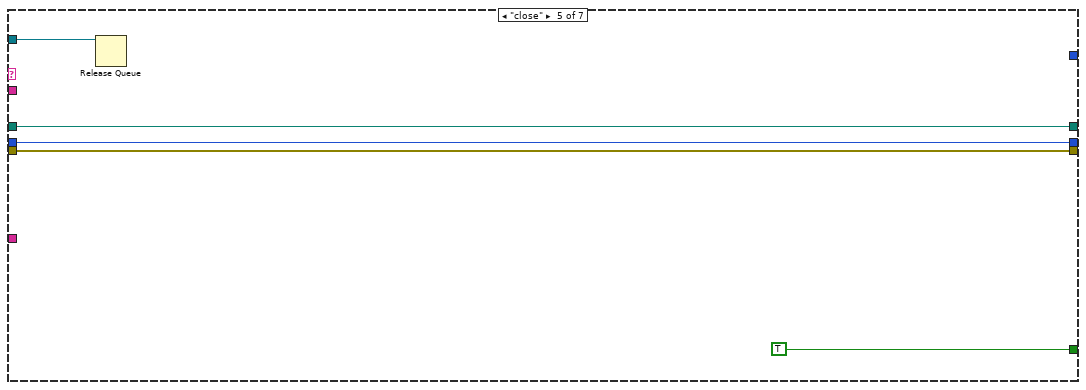
[diagram p13: hidden frame]
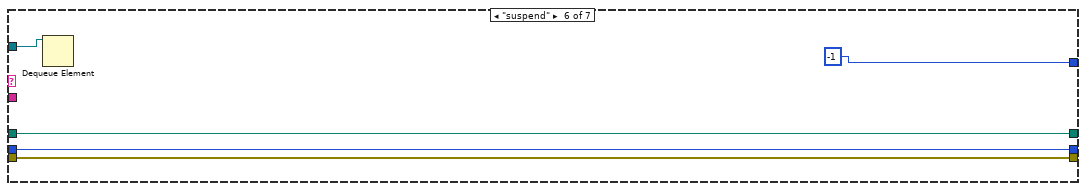
[diagram p14: hidden frame]
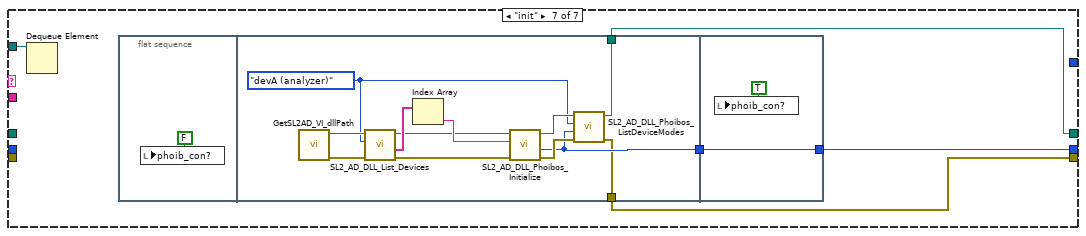
[diagram p15: hidden frame]
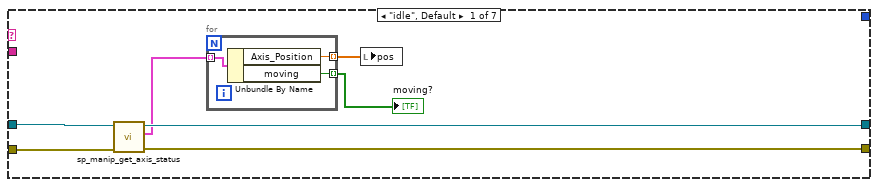
[diagram p16: hidden frame]
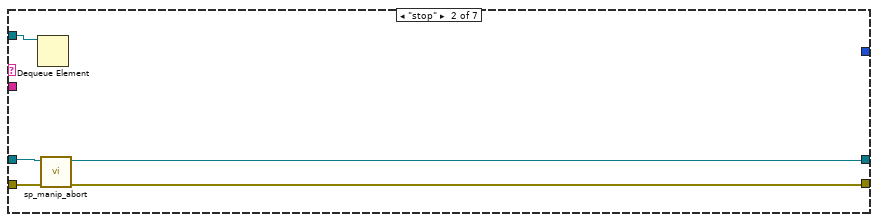
[diagram p17: hidden frame]
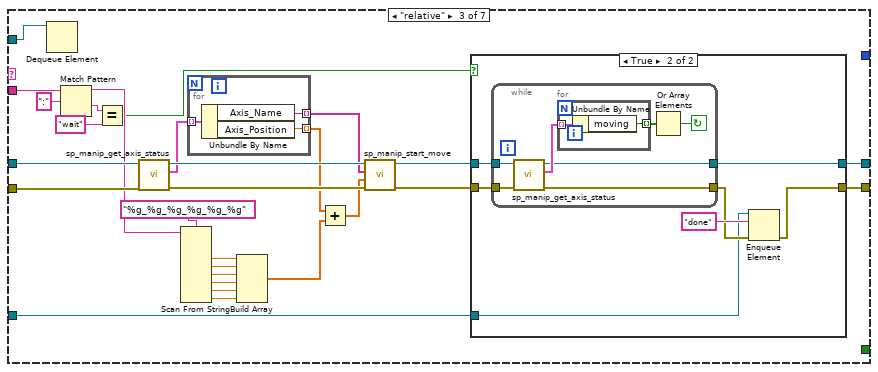
[diagram p18: hidden frame]
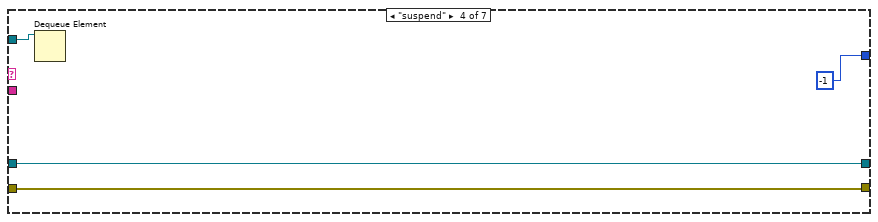
[diagram p20: hidden frame]
diagram:
  w14 = "init" ("name (unnamed)")
  w16 = "" ("name (unnamed)")
  # "scanvector"
  # "imgs"
  # "avg img"
  # "avg"
  # "time"
  # "dark"
  # "Error"
  # "Handle"
  # "memory pointer"
  n1 = Current VI's Path() -> (path=w4:path)
  n2 = Strip Path(path=w4) -> (stripped path=w8:path)  [unwired: 1 out]
  n3 = Strip Path(path=w8) -> (stripped path=w9:path)  [unwired: 1 out]
  n4 = Build Path(base path=w9, name or relative path="runnumber.txt") -> (appended path=w6:path)
  n5 = Obtain Queue(name (unnamed)="dataQ", element data type=dbl[][][] []) -> (queue out=w11:refnum<queue>)  [unwired: 3 in, 2 out]
  n6 = Obtain Queue(name (unnamed)="cam", element data type=w16) -> (queue out=w36:refnum<queue>, error out=w35:errorcluster)  [unwired: 3 in, 1 out]
  n7 = Obtain Queue(name (unnamed)="ESP", element data type=w16) -> (queue out=w33:refnum<queue>, error out=w34:errorcluster)  [unwired: 3 in, 1 out]
  n8 = Obtain Queue(name (unnamed)="manip", element data type=w16) -> (queue out=w30:refnum<queue>, error out=w29:errorcluster)  [unwired: 3 in, 1 out]
  n9 = Obtain Queue(name (unnamed)="phoib", element data type=w16) -> (queue out=w27:refnum<queue>, error out=w28:errorcluster)  [unwired: 3 in, 1 out]
  n10 = Obtain Queue(name (unnamed)="meas", element data type=w16) -> (queue out=w2:refnum<queue>)  [unwired: 3 in, 2 out]
  n11 = Read from Text File(file (use dialog)=w6) -> (text=w7:string)  [unwired: 3 in, 3 out]
  n12 = Enqueue Element(queue=w36, element=w14, error in (no error)=w35) -> (queue out=w10:refnum<queue>)  [unwired: 1 in, 2 out]
  n13 = Enqueue Element(queue=w33, element=w14, error in (no error)=w34) -> (queue out=w13:refnum<queue>)  [unwired: 1 in, 2 out]
  n14 = Enqueue Element(queue=w30, element="suspend" ("name (unnamed)"), error in (no error)=w29) -> (queue out=w3:refnum<queue>)  [unwired: 1 in, 2 out]
  n15 = Enqueue Element(queue=w27, element=w14, error in (no error)=w28) -> (queue out=w24:refnum<queue>)  [unwired: 1 in, 2 out]
  n16 = Decimal String To Number(string=w7) -> (number=w1:i32)  [unwired: 2 in, 1 out]
  n17 = local write "RunNumber"(w1) -> ()
  n18 = while {
    tunnel: w11 -> [w52]
    tunnel: w13 -> [w51]
    tunnel: w10 -> [w50]
    shift-right: [w47] -> _
    shift-left: _ -> [w49]
    shift-right: [w46] -> _
    shift-left: _ -> [w48]
    tunnel: w2 -> [w43]
    tunnel: w3 -> [w38]
    stop <- w39 stop-if-true
    n19 = Preview Queue Element(queue=w43) -> (queue out=w40:refnum<queue>, element=w45:string)  [unwired: 2 in, 2 out]
    n20 = Match Pattern(string=w45, regular expression=":") -> (before substring=w42:string, after substring=w41:string)  [unwired: 1 in, 2 out]
    n21 = case shown="\"delay_chop\"" w42 {
      tunnel: w52 -> [_ _ w86 w245 _ w462 w571]
      tunnel: w51 -> [_ _ w85 w244 _ _ _]
      tunnel: w50 -> [_ _ w84 w243 _ w461 w573]
      tunnel: w49 -> [w54 w58 _ _ w423 w458 w570]
      tunnel: w48 -> [w53 w57 _ _ w421 w457 w569]
      tunnel: [w54 w58 w59 w242 w423 w458 w570] -> w47
      tunnel: [w53 w57 w66 w225 w421 w457 w569] -> w46
      tunnel: w41 -> [_ _ _ _ _ _ _]
      tunnel: w40 -> [w56 _ w75 w234 w425 w456 w572]
      tunnel: [TRUE _ _ _ _ _ _] -> w39
      tunnel: w38 -> [_ _ _ _ _ w460 _]
      frame "close" {
        n22 = Release Queue(queue=w56) -> ()  [unwired: 2 in, 3 out]
      }
      frame "idle", Default {
      }
      frame "GO" {
        n23 = Dequeue Element(queue=w75) -> (queue out=w74:refnum<queue>)  [unwired: 2 in, 3 out]
        n24 = local read "RunNumber"() -> (w81:u16)
        n25 = local read "BasePath"() -> (w80:path)
        n26 = local read "ESP Axis"() -> (w78:i32)
        n27 = local read "ESP_t0"() -> (w64:dbl)
        n28 = Increment(x=w81) -> (x+1=w79:u16)
        n29 = Current VI's Path() -> (path=w82:path)
        n30 = call "2delaypoints.vi"("Offset (mm)"=w64, "delay table [fs]"="delay table [fs]") -> ("delay points [mm]"=w63:dbl[], "delay pointss [fs]"=w61:dbl[])
        n31 = Number To Decimal String(number=w78) -> (decimal integer string=w77:string)  [unwired: 1 in]
        n32 = call "create_opti_path.vi"("RunNumber"=w79, "base path"=w80) -> ("Path"=w71:path)  [unwired: 2 in]
        n33 = call "saverunnumber.vi"("RunNumber"=w79, "VI path"=w82) -> ()  [unwired: 10 in]
        n34 = local write "RunNumber"(w79) -> ()
        n35 = Get Date/Time In Seconds() -> (seconds since 1Jan1904=w60:timestamp)
        n36 = Build Path(base path=w71, name or relative path="info.txt") -> (appended path=w62:path)
        n37 = while {
          tunnel: w63 -> [w123]
          tunnel: w77 -> [w131]
          tunnel: w85 -> [w130]
          tunnel: w86 -> [w129]
          tunnel: w74 -> [w128]
          tunnel: w84 -> [w127]
          tunnel: w71 -> [w126]
          shift-right: [w124] -> w83
          shift-left: dbl[][][] [] -> [w125]
          tunnel: [w122] -> w67
          tunnel: w62 -> [w89]
          tunnel: w61 -> [w88]
          tunnel: w60 -> [w87]
          i -> [w121]
          stop <- w117 stop-if-true
          n38 = for {
            N -> [w153]
            tunnel: w123 -> [w162] mode=indexing
            tunnel: w131 -> [w179]
            tunnel: w130 -> [w178]
            tunnel: w129 -> [w173]
            tunnel: w128 -> [w177]
            tunnel: w127 -> [w176]
            tunnel: w126 -> [w147]
            shift-right: [w137] -> w124
            shift-left: w125 -> [w169]
            tunnel: w121 -> [w146]
            tunnel: w88 -> [w135]
            tunnel: [w135] -> w122
            tunnel: [w159] -> w119
            tunnel: w87 -> [w149]
            tunnel: "delscan_iters" -> [w154]
            i -> [w139]
            stop <- "delscan_abort" stop-if-true
            w181 = ":" ("string")
            # "average data"
            # "init array?"
            n39 = Number To Fractional String(number=w162) -> (F-format string=w171:string)  [unwired: 3 in]
            n40 = property on="delscan_progress" class="Slide (strict)"("Scale.Maximum"=w153) -> ()  [unwired: 2 in, 2 out]
            n41 = Get Date/Time In Seconds() -> (seconds since 1Jan1904=w157:timestamp)
            n42 = call "createFileStruc.vi"("i_iter"=w146, "i_delay"=w139, "meas_path"=w147) -> ("AVG file"=w142:path, "RAW file"=w143:path)  [unwired: 7 in]
            n43 = Concatenate Strings("abs:" ("string"), w179, w181, w171, w181, "wait" ("string")) -> (w184:string)
            n44 = Enqueue Element(queue=w178, element=w184) -> (error out=w182:errorcluster)  [unwired: 2 in, 2 out]
            n45 = Subtract(x=w157, y=w149) -> (x-y=w155:dbl)
            n46 = Equal To 0?(x=w139) -> (x = 0?=w145:bool)
            n47 = Equal To 0?(x=w146) -> (x = 0?=w144:bool)
            n48 = Dequeue Element(queue=w177, error in (no error)=w182) -> (error out=w174:errorcluster)  [unwired: 1 in, 3 out]
            n49 = And(x=w145, y=w144) -> (x .and. y?=w170:bool)
            n50 = Enqueue Element(queue=w176, element="snap", error in (no error)=w174) -> (error out=w172:errorcluster)  [unwired: 1 in, 2 out]
            n51 = Dequeue Element(queue=w173, error in (no error)=w172) -> (element=w165:dbl[][][])  [unwired: 1 in, 3 out]
            n52 = Index Array(array=w165, index (dim 2)=0 ("disabled index (col)")) -> (element=w133:dbl[][])  [unwired: 2 in]
            n53 = Multiply(x=w153, y=w146) -> (x*y=w158:i32)
            n54 = Multiply(x=w153, y=w154) -> (x*y=w152:u32)
            n55 = Array Size(array=w133) -> (size(s)=w166:i32[])
            n56 = Add(x=w158, y=w139) -> (x+y=w156:i32)
            n57 = call-poly <vilib>:"Write Delimited Spreadsheet.vi"("file path (dialog if empty)"=w143, "2D data"=w133) -> ()  [unwired: 12 in, 2 out]
            n58 = Index Array(array=w166) -> (element #1=w164:i32, element #2=w163:i32)  [unwired: 2 in]
            n59 = Divide(x=w155, y=w156) -> (x/y=w151:dbl)
            "time / step" <- w151
            n60 = Multiply(x=w152, y=w151) -> (x*y=w150:dbl)
            n61 = case shown="True" w170 {
              tunnel: w153 -> [_ w192]
              tunnel: [w187 w190] -> w168
              tunnel: w169 -> [w187 _]
              tunnel: w164 -> [_ w189]
              tunnel: w163 -> [_ w188]
              frame False {
              }
              frame True {
                n62 = Initialize Array(0.0 ("element"), w192, w189, w188) -> (w190:dbl[][][])
              }
            }
            n63 = Add(x=w149, y=w150) -> (x+y=→"del_ETA":timestamp)
            n64 = for {
              N: w164 -> [_]
              tunnel: w139 -> [w199]
              shift-right: [w197] -> w137
              shift-left: w168 -> [w200]
              tunnel: w146 -> [w195]
              shift-right: [w194] -> w167
              shift-left: w133 -> [w196]
              tunnel: w163 -> [w193]
              i -> [w198]
              n65 = for {
                N: w193 -> [_]
                tunnel: w199 -> [w207]
                tunnel: w198 -> [w204]
                shift-right: [w206] -> w197
                shift-left: w200 -> [w208]
                tunnel: w195 -> [w202]
                shift-right: [w201] -> w194
                shift-left: w196 -> [w205]
                i -> [w203]
                n66 = in-place {
                  in-place-border: w202 -> [w214]
                  n67 = in-place-array #1(w208, w207, w204, w203) -> (w215:dbl)
                  n68 = in-place-array #2(w205, w204, w203) -> (w212:dbl)
                  n69 = Multiply(x=w215, y=w214) -> (x*y=w213:dbl)
                  n70 = Increment(x=w214) -> (x+1=w210:i32)
                  n71 = Add(x=w213, y=w212) -> (x+y=w211:dbl)
                  n72 = Divide(x=w211, y=w210) -> (x/y=w209:dbl)
                  n73 = in-place-array #1(w209) -> (w206:dbl[][][])  [unwired: 3 out]
                  n74 = in-place-array #2(w209) -> (w201:dbl[][])  [unwired: 2 out]
                }
              }
            }
            n75 = call-poly <vilib>:"Write Delimited Spreadsheet.vi"("file path (dialog if empty)"=w142, "2D data"=w167) -> ()  [unwired: 12 in, 2 out]
            n76 = property on="mainimg" class="IntGraph (strict)"() -> ("CrsrLis"=w138:T4)  [unwired: 2 in, 2 out]
            n77 = call "processData.vi"("Cursor List"=w138, "data in"=w137) -> ("Intensity Chart"=w136:dbl[])  [unwired: 1 in, 2 out]
            n78 = Increment(x=w139) -> (x+1=w140:i32)
            n79 = Bundle("delay pointss [fs]"=w135, "Intensity Chart"=w136) -> (w134:T5)  [unwired: 1 in]
            n80 = flat-sequence {
              tunnel: w134 -> [w186]
              tunnel: [w186] -> w141
              tunnel: w140 -> [w185]
              frame #0 {
                "delscan_progress" <- w185
              }
            }
            n81 = Or(x="delscan_finishIteration", y="delscan_abort") -> (x .or. y?=w159:bool)
            "delscan_pos" <- w162
            "scangraph" <- w141
          }
          n82 = Increment(x=w121) -> (x+1=w120:i32)
          "iteration" <- w120
          n83 = local read "exposure [ms]"() -> (w104:u32)
          n84 = local read "delscan_iters"() -> (w114:u32)
          n85 = local read "ROI Bottom"() -> (w107:i32)
          n86 = property on="Mode" class="Enum (strict)"() -> ("RingText.Text"=w93:string)  [unwired: 2 in, 2 out]
          n87 = property on="VoltageRange" class="Enum (strict)"() -> ("RingText.Text"=w94:string)  [unwired: 2 in, 2 out]
          n88 = local read "cam_dark?"() -> (w91:bool)
          n89 = local read "phoib_I_1"() -> (w95:dbl)
          n90 = local read "phoib_I_2"() -> (w96:dbl)
          n91 = local read "phoib_I_3"() -> (w97:dbl)
          n92 = local read "phoib_I_4"() -> (w98:dbl)
          n93 = local read "phoib_I_5"() -> (w99:dbl)
          n94 = local read "phoib_I_6"() -> (w100:dbl)
          n95 = local read "phoib_I_7"() -> (w101:dbl)
          n96 = local read "phoib_I_8"() -> (w102:dbl)
          n97 = local read "phoib_I_9"() -> (w103:dbl)
          n98 = local read "ROI Right"() -> (w109:i32)
          n99 = local read "averages"() -> (w113:i32)
          n100 = local read "ROI Top"() -> (w108:i32)
          n101 = local read "ROI Left"() -> (w110:i32)
          n102 = local read "binning"() -> (w106:u16)
          n103 = local read "ESP_t0"() -> (w115:dbl)
          n104 = local read "gain"() -> (w90:bool)
          n105 = Boolean To (0,1)(Boolean=w90) -> (0, 1=w105:i16)
          n106 = Boolean To (0,1)(Boolean=w91) -> (0, 1=w111:i16)
          n107 = Format Into String(format string="ScanType:%s\\nAverages:%u\\nRepetitions:%u\\nTimeZero:%f\\nLensMode:%s\\nVoltageRange:%s\\nKineticEnergy:%f\\nPassEnergy:%f\\nCoilCurrent:%f\\nWorkFunction:%f\\nDetectorVoltage:%f\\nScreenVoltage:%f\\nConversionVoltage:%f\\nFocusDisplacement1:%f\\nFocusDisplacement2:%f\\nExposure:%u\\nGain:%u\\nBinning:%u\\nROIbottom:%u\\nROItop:%u\\nROIright:%u\\nROIleft:%u\\nDarkImg:%u\\nStartTime:%<%Y.%m.%d %H:%M:%S>T", initial string=w89, "delay" ("input 1"), w113, w114, w115, w93, w94, w95, w96, w97, w98, w99, w100, w101, w102, w103, w104, w105, w106, w107, w108, w109, w110, w111, w87) -> ()  [unwired: 1 in, 2 out]
          n108 = Less Or Equal?(x="delscan_iters", y=w120) -> (x <= y?=w118:bool)
          n109 = Or(x=w119, y=w118) -> (x .or. y?=w117:bool)
        }
        n110 = Build Path(base path=w71, name or relative path="scanvector.txt") -> (appended path=w68:path)
        n111 = call-poly <vilib>:"Write Delimited Spreadsheet.vi"("file path (dialog if empty)"=w68, "format (%.3f)"="%.6f", "1D data"=w63, "transpose? (no:F)"=TRUE ("transpose? (F)")) -> ()  [unwired: 10 in, 2 out]
        n112 = flat-sequence {
          tunnel: w67 -> [w218]
          tunnel: [w218] -> w66
          frame #0 {
            w217 = u32 1000 ("frequency (Hz)")
            n113 = call <vilib>:"Beep.vi"("use system alert? (T)"=FALSE, "duration (msec)"=w217, "frequency (Hz)"=w217) -> ()  [unwired: 9 in]
          }
        }
        n114 = Build Array(w83) -> (w59:dbl[][][][])
      }
      frame "delay_chop" {
        n115 = local read "delay table [fs]"() -> (w219:string[][])
        n116 = Dequeue Element(queue=w234) -> (queue out=w233:refnum<queue>)  [unwired: 2 in, 3 out]
        n117 = local read "RunNumber"() -> (w240:u16)
        n118 = local read "BasePath"() -> (w239:path)
        n119 = local read "ESP Axis"() -> (w237:i32)
        n120 = local read "ESP_t0"() -> (w224:dbl)
        n121 = Increment(x=w240) -> (x+1=w238:u16)
        n122 = Current VI's Path() -> (path=w241:path)
        n123 = call "2delaypoints.vi"("Offset (mm)"=w224, "delay table [fs]"=w219) -> ("delay points [mm]"=w223:dbl[], "delay pointss [fs]"=w221:dbl[])
        n124 = Number To Decimal String(number=w237) -> (decimal integer string=w236:string)  [unwired: 1 in]
        n125 = call "create_opti_path.vi"("RunNumber"=w238, "base path"=w239) -> ("Path"=w230:path)  [unwired: 2 in]
        n126 = call "saverunnumber.vi"("RunNumber"=w238, "VI path"=w241) -> ()  [unwired: 10 in]
        n127 = local write "RunNumber"(w238) -> ()
        n128 = Get Date/Time In Seconds() -> (seconds since 1Jan1904=w220:timestamp)
        n129 = Build Path(base path=w230, name or relative path="info.txt") -> (appended path=w222:path)
        n130 = while {
          tunnel: w223 -> [w282]
          tunnel: w236 -> [w290]
          tunnel: w244 -> [w289]
          tunnel: w245 -> [w288]
          tunnel: w233 -> [w287]
          tunnel: w243 -> [w286]
          tunnel: w230 -> [w285]
          shift-right: [w283] -> w242
          shift-left: dbl[][][][] [] -> [w284]
          tunnel: [w281] -> w226
          tunnel: w222 -> [w250]
          tunnel: w221 -> [w249]
          tunnel: w220 -> [w248]
          i -> [w280]
          stop <- w277 stop-if-true
          n131 = Increment(x=w280) -> (x+1=w247:i32)
          n132 = local read "exposure [ms]"() -> (w265:u32)
          n133 = local read "delscan_iters"() -> (w275:u32)
          n134 = local read "ROI Bottom"() -> (w268:i32)
          n135 = property on="Mode" class="Enum (strict)"() -> ("RingText.Text"=w254:string)  [unwired: 2 in, 2 out]
          n136 = property on="VoltageRange" class="Enum (strict)"() -> ("RingText.Text"=w255:string)  [unwired: 2 in, 2 out]
          n137 = local read "cam_dark?"() -> (w252:bool)
          n138 = local write "iteration"(w247) -> ()
          n139 = local read "phoib_I_1"() -> (w256:dbl)
          n140 = local read "phoib_I_2"() -> (w257:dbl)
          n141 = local read "phoib_I_3"() -> (w258:dbl)
          n142 = local read "phoib_I_4"() -> (w259:dbl)
          n143 = local read "phoib_I_5"() -> (w260:dbl)
          n144 = local read "phoib_I_6"() -> (w261:dbl)
          n145 = local read "phoib_I_7"() -> (w262:dbl)
          n146 = local read "phoib_I_8"() -> (w263:dbl)
          n147 = local read "phoib_I_9"() -> (w264:dbl)
          n148 = local read "ROI Right"() -> (w270:i32)
          n149 = local read "averages"() -> (w274:i32)
          n150 = local read "ROI Top"() -> (w269:i32)
          n151 = local read "ROI Left"() -> (w271:i32)
          n152 = local read "binning"() -> (w267:u16)
          n153 = local read "ESP_t0"() -> (w276:dbl)
          n154 = local read "gain"() -> (w251:bool)
          n155 = Boolean To (0,1)(Boolean=w251) -> (0, 1=w266:i16)
          n156 = Boolean To (0,1)(Boolean=w252) -> (0, 1=w272:i16)
          n157 = local read "delscan_iters"() -> (w246:u32)
          n158 = for {
            N -> [w335]
            tunnel: w282 -> [w332] mode=indexing
            tunnel: w290 -> [w366]
            tunnel: w289 -> [w365]
            tunnel: w288 -> [w360]
            tunnel: w287 -> [w364]
            tunnel: w286 -> [w363]
            tunnel: w285 -> [w342]
            shift-right: [w314] -> w283
            shift-left: w284 -> [w356]
            tunnel: w280 -> [w341]
            tunnel: w249 -> [w310]
            tunnel: [w310] -> w281
            tunnel: [w351] -> w279
            tunnel: w248 -> [w343]
            tunnel: w246 -> [w346]
            i -> [w337]
            stop <- "delscan_abort 2" stop-if-true
            (unwired) 1 ("disabled index (col)")
            w368 = ":" ("string")
            # "init array?"
            n159 = local write "delscan_pos"(w332) -> ()
            n160 = Number To Fractional String(number=w332) -> (F-format string=w358:string)  [unwired: 3 in]
            n161 = Get Date/Time In Seconds() -> (seconds since 1Jan1904=w349:timestamp)
            n162 = call "createFileStruc.vi"("i_iter"=w341, "i_delay"=w337, "meas_path"=w342) -> ("AVG file"=w297:path, "RAW file"=w304:path)  [unwired: 7 in]
            n163 = property on="delscan_progress" class="Slide (strict)"("Scale.Maximum"=w335) -> ()  [unwired: 2 in, 2 out]
            n164 = Concatenate Strings("abs:" ("string"), w366, w368, w358, w368, "wait" ("string")) -> (w371:string)
            n165 = Enqueue Element(queue=w365, element=w371) -> (error out=w369:errorcluster)  [unwired: 2 in, 2 out]
            n166 = Subtract(x=w349, y=w343) -> (x-y=w347:dbl)
            n167 = Equal To 0?(x=w337) -> (x = 0?=w340:bool)
            n168 = Equal To 0?(x=w341) -> (x = 0?=w339:bool)
            n169 = Dequeue Element(queue=w364, error in (no error)=w369) -> (error out=w361:errorcluster)  [unwired: 1 in, 3 out]
            n170 = And(x=w340, y=w339) -> (x .and. y?=w357:bool)
            n171 = Enqueue Element(queue=w363, element="snap", error in (no error)=w361) -> (error out=w359:errorcluster)  [unwired: 1 in, 2 out]
            n172 = Strip Path(path=w304) -> (stripped path=w303:path, name=w300:string)
            n173 = Dequeue Element(queue=w360, error in (no error)=w359) -> (element=w326:dbl[][][])  [unwired: 1 in, 3 out]
            n174 = Concatenate Strings(w300, ".l" ("name or relative path")) -> (w298:string)
            n175 = Concatenate Strings(w300, ".nl" ("name or relative path")) -> (w301:string)
            n176 = Multiply(x=w335, y=w341) -> (x*y=w350:i32)
            n177 = Multiply(x=w335, y=w346) -> (x*y=w345:u32)
            n178 = Index Array(array=w326, index (dim 2)=1 ("disabled index (col)")) -> (element=w329:dbl[][])  [unwired: 2 in]
            n179 = Build Path(base path=w303, name or relative path=w298) -> (appended path=w324:path)
            n180 = Build Path(base path=w303, name or relative path=w301) -> (appended path=w323:path)
            n181 = Array Size(array=w326) -> (size(s)=w354:i32[])
            n182 = Index Array(array=w326, index (dim 2)=0 ("disabled index (col)")) -> (element=w327:dbl[][])  [unwired: 2 in]
            n183 = Add(x=w350, y=w337) -> (x+y=w348:i32)
            n184 = Index Array(array=w354) -> (element #1=w353:i32, element #2=w352:i32, element #3=w305:i32)  [unwired: 3 in]
            n185 = Divide(x=w347, y=w348) -> (x/y=w333:dbl)
            n186 = call-poly <vilib>:"Write Delimited Spreadsheet.vi"("file path (dialog if empty)"=w323, "2D data"=w329) -> ()  [unwired: 12 in, 2 out]
            n187 = call-poly <vilib>:"Write Delimited Spreadsheet.vi"("file path (dialog if empty)"=w324, "2D data"=w327) -> ()  [unwired: 12 in, 2 out]
            n188 = Multiply(x=w345, y=w333) -> (x*y=w344:dbl)
            n189 = case shown="True" w357 {
              tunnel: w335 -> [_ w414]
              tunnel: [w408 w412] -> w355
              tunnel: w356 -> [w408 _]
              tunnel: w353 -> [_ w411]
              tunnel: w352 -> [_ w410]
              tunnel: w305 -> [_ w409]
              frame False {
              }
              frame True {
                n190 = Initialize Array(0.0 ("element"), w414, w411, w410, w409) -> (w412:dbl[][][][])
              }
            }
            n191 = Add(x=w343, y=w344) -> (x+y=w334:timestamp)
            n192 = local write "del_ETA"(w334) -> ()
            n193 = local write "time / step"(w333) -> ()
            n194 = for {
              N: w305 -> [_]
              tunnel: w353 -> [w377]
              tunnel: w352 -> [w376]
              tunnel: w341 -> [w375]
              tunnel: w337 -> [w374]
              shift-right: [w373] -> w314
              shift-left: w355 -> [w380]
              shift-right: [w379] -> w319
              shift-left: w326 -> [w378]
              i -> [w372]
              # "average data"
              n195 = for {
                N: w377 -> [_]
                tunnel: w374 -> [w388]
                shift-right: [w386] -> w373
                shift-left: w380 -> [w389]
                tunnel: w375 -> [w384]
                shift-right: [w383] -> w379
                shift-left: w378 -> [w385]
                tunnel: w376 -> [w382]
                tunnel: w372 -> [w381]
                i -> [w387]
                n196 = for {
                  N: w382 -> [_]
                  tunnel: w388 -> [w397]
                  tunnel: w387 -> [w394]
                  shift-right: [w396] -> w386
                  shift-left: w389 -> [w398]
                  tunnel: w384 -> [w392]
                  shift-right: [w391] -> w383
                  shift-left: w385 -> [w395]
                  tunnel: w381 -> [w390]
                  i -> [w393]
                  n197 = in-place {
                    in-place-border: w392 -> [w404]
                    n198 = in-place-array #3(w398, w397, w394, w393, w390) -> (w405:dbl)
                    n199 = in-place-array #4(w395, w394, w393, w390) -> (w402:dbl)
                    n200 = Multiply(x=w405, y=w404) -> (x*y=w403:dbl)
                    n201 = Increment(x=w404) -> (x+1=w400:i32)
                    n202 = Add(x=w403, y=w402) -> (x+y=w401:dbl)
                    n203 = Divide(x=w401, y=w400) -> (x/y=w399:dbl)
                    n204 = in-place-array #3(w399) -> (w396:dbl[][][][])  [unwired: 4 out]
                    n205 = in-place-array #4(w399) -> (w391:dbl[][][])  [unwired: 3 out]
                  }
                }
              }
            }
            n206 = Strip Path(path=w297) -> (stripped path=w296:path, name=w295:string)
            n207 = Concatenate Strings(w295, ".l" ("name or relative path")) -> (w292:string)
            n208 = Concatenate Strings(w295, ".nl" ("name or relative path")) -> (w291:string)
            n209 = Build Path(base path=w296, name or relative path=w292) -> (appended path=w322:path)
            n210 = Build Path(base path=w296, name or relative path=w291) -> (appended path=w317:path)
            n211 = Index Array(array=w319, index (dim 2)=0 ("disabled index (col)")) -> (element=w320:dbl[][])  [unwired: 2 in]
            n212 = Index Array(array=w319) -> (element=w318:dbl[][])  [unwired: 3 in]
            n213 = call-poly <vilib>:"Write Delimited Spreadsheet.vi"("file path (dialog if empty)"=w322, "2D data"=w320) -> ()  [unwired: 12 in, 2 out]
            n214 = call-poly <vilib>:"Write Delimited Spreadsheet.vi"("file path (dialog if empty)"=w317, "2D data"=w318) -> ()  [unwired: 12 in, 2 out]
            n215 = Index Array(array=w314, index (dim 3)=1 ("disabled index (col)")) -> (element=w312:dbl[][][])  [unwired: 3 in]
            n216 = Index Array(array=w314, index (dim 3)=0 ("disabled index (col)")) -> (element=w315:dbl[][][])  [unwired: 3 in]
            n217 = Increment(x=w337) -> (x+1=w338:i32)
            n218 = property on="mainimg" class="IntGraph (strict)"() -> ("CrsrLis"=w311:T4)  [unwired: 2 in, 2 out]
            n219 = call "processData.vi"("Cursor List"=w311, "data in"=w315) -> ("Intensity Chart"=w336:dbl[])  [unwired: 1 in, 2 out]
            n220 = call "processData.vi"("Cursor List"=w311, "data in"=w312) -> ("Intensity Chart"=w309:dbl[])  [unwired: 1 in, 2 out]
            n221 = Bundle("delay pointss [fs]"=w310, "Intensity Chart"=w336) -> (w308:T5)  [unwired: 1 in]
            n222 = Bundle("delay pointss [fs]"=w310, "Intensity Chart"=w309) -> (w307:T5)  [unwired: 1 in]
            n223 = flat-sequence {
              tunnel: w338 -> [w407]
              tunnel: w308 -> [w406]
              tunnel: w307 -> [_]
              tunnel: [w406] -> w306
              frame #0 {
                n224 = local write "delscan_progress"(w407) -> ()
              }
            }
            n225 = Or(x="delscan_finishIteration 2", y="delscan_abort 2") -> (x .or. y?=w351:bool)
            n226 = local write "scangraph"(w306) -> ()
          }
          n227 = Format Into String(format string="ScanType:%s\\nAverages:%u\\nRepetitions:%u\\nTimeZero:%f\\nLensMode:%s\\nVoltageRange:%s\\nKineticEnergy:%f\\nPassEnergy:%f\\nCoilCurrent:%f\\nWorkFunction:%f\\nDetectorVoltage:%f\\nScreenVoltage:%f\\nConversionVoltage:%f\\nFocusDisplacement1:%f\\nFocusDisplacement2:%f\\nExposure:%u\\nGain:%u\\nBinning:%u\\nROIbottom:%u\\nROItop:%u\\nROIright:%u\\nROIleft:%u\\nDarkImg:%u\\nStartTime:%<%Y.%m.%d %H:%M:%S>T", initial string=w250, "delay" ("input 1"), w274, w275, w276, w254, w255, w256, w257, w258, w259, w260, w261, w262, w263, w264, w265, w266, w267, w268, w269, w270, w271, w272, w248) -> ()  [unwired: 1 in, 2 out]
          n228 = Less Or Equal?(x=w246, y=w247) -> (x <= y?=w278:bool)
          n229 = Or(x=w279, y=w278) -> (x .or. y?=w277:bool)
        }
        n230 = Build Path(base path=w230, name or relative path="scanvector.txt") -> (appended path=w227:path)
        n231 = call-poly <vilib>:"Write Delimited Spreadsheet.vi"("file path (dialog if empty)"=w227, "format (%.3f)"="%.6f", "1D data"=w223, "transpose? (no:F)"=TRUE ("transpose? (F)")) -> ()  [unwired: 10 in, 2 out]
        n232 = flat-sequence {
          tunnel: w226 -> [w417]
          tunnel: [w417] -> w225
          frame #0 {
            w416 = u32 1000 ("frequency (Hz)")
            n233 = call <vilib>:"Beep.vi"("use system alert? (T)"=FALSE, "duration (msec)"=w416, "frequency (Hz)"=w416) -> ()  [unwired: 9 in]
          }
        }
      }
      frame "refresh" {
        n234 = Dequeue Element(queue=w425) -> ()  [unwired: 2 in, 4 out]
        n235 = property on="mainimg" class="IntGraph (strict)"() -> ("CrsrLis"=w424:T4)  [unwired: 2 in, 2 out]
        n236 = Index Array(array=w423, index (dim 3)=0 ("disabled index (col)")) -> (element=w419:dbl[][][])  [unwired: 3 in]
        n237 = call "processData.vi"("Cursor List"=w424, "data in"=w419) -> ("Intensity Chart"=w422:dbl[])  [unwired: 1 in, 2 out]
        n238 = Bundle("delay pointss [fs]"=w421, "Intensity Chart"=w422) -> (w420:T5)  [unwired: 1 in]
        n239 = local write "scangraph"(w420) -> ()
      }
      frame "manip" {
        n240 = Dequeue Element(queue=w456) -> (queue out=w455:refnum<queue>)  [unwired: 2 in, 3 out]
        n241 = local read "RunNumber"() -> (w464:u16)
        n242 = local read "BasePath"() -> (w465:path)
        n243 = property on="delscan_progress 2" class="Slide (strict)"("Scale.Maximum"="manip_scan_steps") -> ()  [unwired: 2 in, 2 out]
        n244 = Index Array(array="manip_scan_delta") -> (element #1=w477:dbl, element #2=w476:dbl, element #3=w475:dbl, element #4=w474:dbl, element #5=w473:dbl, element #6=w472:dbl)  [unwired: 6 in]
        n245 = Increment(x=w464) -> (x+1=w466:u16)
        n246 = Current VI's Path() -> (path=w463:path)
        n247 = Format Into String(format string="%g_%g_%g_%g_%g_%g", w477, w476, w475, w474, w473, w472) -> (resulting string=w470:string)  [unwired: 2 in, 1 out]
        n248 = property on="Mode" class="Enum (strict)"() -> ("RingText.Text"=w450:string)  [unwired: 2 in, 2 out]
        n249 = property on="VoltageRange" class="Enum (strict)"() -> ("RingText.Text"=w449:string)  [unwired: 2 in, 2 out]
        n250 = call "saverunnumber.vi"("RunNumber"=w466, "VI path"=w463) -> ()  [unwired: 10 in]
        n251 = local write "RunNumber"(w466) -> ()
        n252 = call "create_opti_path.vi"("RunNumber"=w466, "base path"=w465) -> ("Path"=w429:path)  [unwired: 2 in]
        n253 = local read "exposure [ms]"() -> (w439:u32)
        n254 = Build Path(base path=w429, name or relative path="info.txt") -> (appended path=w428:path)
        n255 = Concatenate Strings("relative:" ("string"), w470, ":wait" ("string")) -> (w479:string)
        n256 = local read "ROI Bottom"() -> (w436:i32)
        n257 = local read "cam_dark?"() -> (w453:bool)
        n258 = local read "phoib_I_1"() -> (w448:dbl)
        n259 = local read "phoib_I_2"() -> (w447:dbl)
        n260 = local read "phoib_I_3"() -> (w446:dbl)
        n261 = local read "phoib_I_4"() -> (w445:dbl)
        n262 = local read "phoib_I_5"() -> (w444:dbl)
        n263 = local read "phoib_I_6"() -> (w443:dbl)
        n264 = local read "phoib_I_7"() -> (w442:dbl)
        n265 = local read "phoib_I_8"() -> (w441:dbl)
        n266 = local read "phoib_I_9"() -> (w440:dbl)
        n267 = local read "ROI Right"() -> (w434:i32)
        n268 = local read "averages"() -> (w451:i32)
        n269 = local read "ROI Top"() -> (w435:i32)
        n270 = local read "ROI Left"() -> (w433:i32)
        n271 = local read "binning"() -> (w437:u16)
        n272 = local read "gain"() -> (w454:bool)
        n273 = Get Date/Time In Seconds() -> (seconds since 1Jan1904=w431:timestamp)
        n274 = Build Path(base path=w429, name or relative path="scanvector.txt") -> (appended path=w480:path)
        n275 = for {
          N: 1 -> [_]
          tunnel: w462 -> [w495]
          tunnel: w429 -> [w494]
          tunnel: w480 -> [w487]
          tunnel: "manip_scan_steps" -> [w486]
          tunnel: w479 -> [w485]
          tunnel: w460 -> [w484]
          tunnel: w455 -> [w483]
          tunnel: w461 -> [w482]
          tunnel: "manip_scan_delta" -> [w481]
          i -> [w489]
          n276 = Add(x=w489, y=1000) -> (x+y=w492:i32)
          n277 = Number To Decimal String(number=w492) -> (decimal integer string=w491:string)  [unwired: 1 in]
          n278 = String Subset(string=w491, offset (0)=1) -> (substring=w488:string)  [unwired: 1 in]
          n279 = for {
            N: w486 -> [_]
            tunnel: w495 -> [w520]
            tunnel: w494 -> [w517]
            tunnel: w488 -> [w511]
            tunnel: w487 -> [w513]
            tunnel: w485 -> [w508]
            tunnel: w484 -> [w507]
            tunnel: w483 -> [w506]
            tunnel: w482 -> [w505]
            tunnel: w481 -> [w503]
            i -> [w498]
            stop <- "abort" stop-if-true
            n280 = Increment(x=w498) -> (x+1=→"delscan_progress 2":i32)
            n281 = Multiply(x=w503, y=w498) -> (x*y=w502:dbl[])
            n282 = Enqueue Element(queue=w507, element=w508) -> (error out=w509:errorcluster)  [unwired: 2 in, 2 out]
            n283 = Add(x=w498, y=10000) -> (x+y=w526:i32)
            n284 = Dequeue Element(queue=w506, error in (no error)=w509) -> (error out=w504:errorcluster)  [unwired: 1 in, 3 out]
            n285 = Number To Decimal String(number=w526) -> (decimal integer string=w525:string)  [unwired: 1 in]
            n286 = String Subset(string=w525, offset (0)=1) -> (substring=w510:string)  [unwired: 1 in]
            n287 = Enqueue Element(queue=w505, element="snap", error in (no error)=w504) -> (error out=w519:errorcluster)  [unwired: 1 in, 2 out]
            n288 = Concatenate Strings("RAW\\" ("string"), w511, "_" ("string"), w510, ".tsv" ("string")) -> (w516:string)
            n289 = Dequeue Element(queue=w520, error in (no error)=w519) -> (element=w515:dbl[][][])  [unwired: 1 in, 3 out]
            n290 = Build Path(base path=w517, name or relative path=w516) -> (appended path=w518:path)
            n291 = Index Array(array=w515, index (dim 2)=0 ("disabled index (col)")) -> (element=w497:dbl[][])  [unwired: 2 in]
            n292 = call-poly <vilib>:"Write Delimited Spreadsheet.vi"("file path (dialog if empty)"=w518, "2D data"=w497) -> ()  [unwired: 12 in, 2 out]
            n293 = call-poly <vilib>:"Write Delimited Spreadsheet.vi"("file path (dialog if empty)"=w513, "1D data"=w502, "append to file? (new file:F)"=TRUE ("append to file? (F)"), "transpose? (no:F)"=FALSE ("transpose? (F)")) -> ()  [unwired: 10 in, 2 out]
          }
        }
        n294 = Boolean To (0,1)(Boolean=w454) -> (0, 1=w438:i16)
        n295 = Boolean To (0,1)(Boolean=w453) -> (0, 1=w432:i16)
        n296 = Format Into String(format string="ScanType:%s\\nAverages:%u\\nMode:%s\\nVoltageRange:%s\\nKineticEnergy:%f\\nPassEnergy:%f\\nCoilCurrent:%f\\nWorkFunction:%f\\nDetectorVoltage:%f\\nScreenVoltage:%f\\nConversionVoltage:%f\\nFocusDisplacement1:%f\\nFocusDisplacement2:%f\\nExposure:%u\\nGain:%u\\nBinning:%u\\nROIbottom:%u\\nROItop:%u\\nROIright:%u\\nROIleft:%u\\nDarkImg:%u\\nStartTime:%<%Y.%m.%d %H:%M:%S>T", initial string=w428, "manipulator" ("input 1"), w451, w450, w449, w448, w447, w446, w445, w444, w443, w442, w441, w440, w439, w438, w437, w436, w435, w434, w433, w432, w431) -> ()  [unwired: 1 in, 2 out]
      }
      frame "single" {
        n297 = Dequeue Element(queue=w572) -> ()  [unwired: 2 in, 4 out]
        n298 = property on="Mode" class="Enum (strict)"() -> ("RingText.Text"=w557:string)  [unwired: 2 in, 2 out]
        n299 = property on="VoltageRange" class="Enum (strict)"() -> ("RingText.Text"=w556:string)  [unwired: 2 in, 2 out]
        n300 = local read "RunNumber"() -> (w563:u16)
        n301 = local read "BasePath"() -> (w564:path)
        n302 = local read "exposure [ms]"() -> (w546:u32)
        n303 = local read "ROI Bottom"() -> (w543:i32)
        n304 = local read "cam_dark?"() -> (w560:bool)
        n305 = local read "phoib_I_1"() -> (w555:dbl)
        n306 = local read "phoib_I_2"() -> (w554:dbl)
        n307 = local read "phoib_I_3"() -> (w553:dbl)
        n308 = local read "phoib_I_4"() -> (w552:dbl)
        n309 = local read "phoib_I_5"() -> (w551:dbl)
        n310 = local read "phoib_I_6"() -> (w550:dbl)
        n311 = local read "phoib_I_7"() -> (w549:dbl)
        n312 = local read "phoib_I_8"() -> (w548:dbl)
        n313 = local read "phoib_I_9"() -> (w547:dbl)
        n314 = local read "ROI Right"() -> (w541:i32)
        n315 = local read "ESP_pos"() -> (w530:dbl)
        n316 = local read "averages"() -> (w558:i32)
        n317 = local read "ROI Top"() -> (w542:i32)
        n318 = local read "ROI Left"() -> (w540:i32)
        n319 = local read "binning"() -> (w544:u16)
        n320 = local read "ESP_t0"() -> (w531:dbl)
        n321 = Increment(x=w563) -> (x+1=w565:u16)
        n322 = Current VI's Path() -> (path=w562:path)
        n323 = local read "gain"() -> (w561:bool)
        n324 = Get Date/Time In Seconds() -> (seconds since 1Jan1904=w538:timestamp)
        n325 = call "saverunnumber.vi"("RunNumber"=w565, "VI path"=w562) -> ()  [unwired: 10 in]
        n326 = local write "RunNumber"(w565) -> ()
        n327 = call "create_opti_path.vi"("RunNumber"=w565, "base path"=w564) -> ("Path"=w535:path)  [unwired: 2 in]
        n328 = Boolean To (0,1)(Boolean=w561) -> (0, 1=w545:i16)
        n329 = Boolean To (0,1)(Boolean=w560) -> (0, 1=w539:i16)
        n330 = Build Path(base path=w535, name or relative path="info.txt") -> (appended path=w533:path)
        n331 = Format Into String(format string="ScanType=%s\\nDelayPosition=%.6f\\nTimeZero=%.6f\\nAverages=%u\\nLensMode=%s\\nVoltageRange=%s\\nKineticEnergy=%f\\nPassEnergy=%f\\nCoilCurrent=%f\\nWorkFunction=%f\\nDetectorVoltage=%f\\nScreenVoltage=%f\\nConversionVoltage=%f\\nFocusDisplacement1=%f\\nFocusDisplacement2=%f\\nExposure=%u\\nGain=%u\\nBinning=%u\\nROIbottom=%u\\nROItop=%u\\nROIright=%u\\nROIleft=%u\\nDarkImg=%u\\nStartTime=%<%Y.%m.%d %H:%M:%S>T", initial string=w533, "single" ("input 1"), w530, w531, w558, w557, w556, w555, w554, w553, w552, w551, w550, w549, w548, w547, w546, w545, w544, w543, w542, w541, w540, w539, w538) -> ()  [unwired: 1 in, 2 out]
        n332 = Build Path(base path=w535, name or relative path="AVG\\000.tsv") -> (appended path=w536:path)
        n333 = Enqueue Element(queue=w573, element="snap" ("string")) -> (error out=w567:errorcluster)  [unwired: 2 in, 2 out]
        n334 = Dequeue Element(queue=w571, error in (no error)=w567) -> (element=w566:dbl[][][])  [unwired: 1 in, 3 out]
        n335 = Index Array(array=w566, index (dim 2)=0 ("disabled index (col)")) -> (element=w529:dbl[][])  [unwired: 2 in]
        n336 = call-poly <vilib>:"Write Delimited Spreadsheet.vi"("file path (dialog if empty)"=w536, "2D data"=w529) -> ()  [unwired: 12 in, 2 out]
      }
    }
  }
  n337 = while {
    tunnel: w10 -> [w600]
    shift-right: [w594] -> _
    shift-left: _ -> [w593]
    shift-right: [w592] -> _
    shift-left: _ -> [w590]
    shift-right: [w591] -> _
    shift-left: _ -> [w589]
    shift-right: [w586] -> _
    shift-left: 0 -> [w587]
    shift-right: [w585] -> _
    shift-left: _ -> [w584]
    shift-right: [w583] -> _
    shift-left: _ -> [w582]
    tunnel: w11 -> [w581]
    shift-right: [w580] -> _
    shift-left: _ -> [w579]
    shift-right: [w577] -> _
    shift-left: _ -> [w576]
    shift-right: [w575] -> _
    shift-left: _ -> [w574]
    i -> [w578]
    stop <- w588 stop-if-true
    # "cam"
    n338 = Preview Queue Element(queue=w600, timeout in ms (-1)=w587) -> (queue out=w599:refnum<queue>, element=w598:string)  [unwired: 1 in, 2 out]
    n339 = Match Pattern(string=w598, regular expression=":") -> (before substring=w595:string, after substring=w596:string)  [unwired: 1 in, 2 out]
    n340 = case shown="\"snap\"" w595 {
      tunnel: w599 -> [w613 w645 w675 w715 w728 _ w816 w855 w965]
      tunnel: w596 -> [_ _ _ _ _ _ _ _ _]
      tunnel: [w607 w632 w671 w714 w726 w769 w813 w840 w963] -> w594
      tunnel: w593 -> [_ _ w671 w714 w726 w769 w813 w840 w963]
      tunnel: [w612 w646 w681 u64 0 ("Hout") w725 w773 w814 w850 w962] -> w592
      tunnel: [w614 w647 w682 w711 w724 w774 w815 w841 w961] -> w591
      tunnel: w590 -> [_ w649 w685 w713 w725 w776 w818 w852 w962]
      tunnel: w589 -> [_ w648 w677 _ w724 w775 w817 w851 w961]
      tunnel: [_ _ _ _ TRUE _ _ _ _] -> w588
      tunnel: [_ _ _ _ _ _ _ _ -1] -> w586
      tunnel: [w606 w633 w676 _ _ w783 _ _ _] -> w585
      tunnel: w584 -> [w606 w633 w676 _ _ w782 _ _ _]
      tunnel: [w607 w635 w678 w709 w723 w778 w807 w853 w960] -> w583
      tunnel: w582 -> [_ w635 w678 w709 w723 w778 _ w853 w960]
      tunnel: w581 -> [_ _ _ _ _ _ _ w844 _]
      tunnel: [w604 w630 w680 w708 w721 w736 w804 w847 w959] -> w580
      tunnel: w579 -> [w604 w630 w680 w708 w721 w771 w804 w847 w959]
      tunnel: w578 -> [_ _ _ _ _ w744 _ _ _]
      tunnel: [w605 w631 w679 w707 w722 w770 w803 w846 w958] -> w577
      tunnel: w576 -> [w605 w631 w679 w707 w722 w743 w803 w846 w958]
      tunnel: [w601 w627 w665 refnum<k21> refnum ("task out") w720 w729 w802 w837 w957] -> w575
      tunnel: w574 -> [_ w627 w666 w706 w720 w729 w802 w838 w957]
      frame "init" {
        w602 = 10106 items=["Default"=-1, "RSE"=10083, "NRSE"=10078, "Differential"=10106, "Pseudodifferential"=12529] ("input terminal configuration")
        w607 = u16[][] []
        n341 = flat-sequence {
          tunnel: [w616] -> w611
          tunnel: [w617] -> w610
          tunnel: [w625] -> w612
          tunnel: [w626] -> w614
          tunnel: w611 -> [w626]
          tunnel: w610 -> [w625]
          frame #0 {
            n342 = local write "cam_con?"(FALSE ("cam_con?")) -> ()
          }
          frame #1 {
            n343 = call "SCInitBoard.vi"("boardnr"="board number") -> ("Hout"=w620:u32, "error out"=w621:errorcluster)  [unwired: 1 in, 1 out]
            n344 = call "SCSetupCamera.vi"("Handle"=w620, "error in (no error)"=w621) -> ("Hout"=w622:u64, "error out"=w623:errorcluster)  [unwired: 1 out]
            n345 = call "SCStopCOC.vi"("error in (no error)"=w623, "Stop mode"=0, "Handle"=w622) -> ("error out"=w616:errorcluster, "Hout"=w617:u64)
          }
          frame #2 {
            n346 = local write "cam_con?"(TRUE ("cam_con?")) -> ()
          }
        }
        n347 = Dequeue Element(queue=w613) -> (queue out=w609:refnum<queue>)  [unwired: 2 in, 3 out]
        n348 = Enqueue Element At Opposite End(queue=w609, element="set") -> ()  [unwired: 2 in, 3 out]
        n349 = call-poly <vilib>:"DAQmx Create Virtual Channel.vi"("input terminal configuration"=w602, "physical channels"=tag "Dev2/ai0") -> ("task out"=w601:refnum<k21>)  [unwired: 12 in, 1 out]
      }
      frame "set" {
        n350 = Dequeue Element(queue=w645) -> ()  [unwired: 2 in, 4 out]
        n351 = call "SCStopCOC.vi"("error in (no error)"=w648, "Stop mode"=0, "Handle"=w649) -> ("error out"=w664:errorcluster, "Hout"=w663:u64)
        n352 = Bundle By Name(cluster=cluster{"Delay":dbl, "Exposure ":dbl} {"Delay"=0.0, "Exposure "=0.0} ("Delay and exposure"), "Exposure"="exposure [ms]") -> (w642:cluster{"Delay":dbl, "Exposure ":dbl})
        n353 = Bundle By Name(cluster=T6 {"Camera type"=0, "Operating mode\nHP & QE / HS & DiCam Pro "=0, "Frame trigger \n(High Performance and QE only)"=0, "Sequence trigger"=0, "Low Light\n(QE only)"=FALSE, "Gain"=FALSE, "Horzontal\nbinning"=0, "Vertical\nbinning "=0, "ROI Left"=1, "ROI Right"=20, "ROI Top"=1, "ROI Bottom"=15} ("Camera controls"), "Operating mode\nHP & QE / HS & DiCam Pro"="Operating mode\nHP & QE / HS & DiCam Pro", "Horzontal\nbinning"="binning", "Vertical\nbinning"="binning", "ROI Left"="ROI Left", "ROI Right"="ROI Right", "ROI Top"="ROI Top", "ROI Bottom"="ROI Bottom", "Gain"="gain", "Frame trigger \n(High Performance and QE only)"="Frame trigger \n(High Performance and QE only)") -> (w659:T6)
        n354 = call "New delay and exposure forma.vi"("Operating mode\nHP & QE / HS & DiCam Pro"="Operating mode\nHP & QE / HS & DiCam Pro", "Delay and exposure"=w642) -> ("Output table"=w660:string)  [unwired: 3 in]
        n355 = call "SCSetCoC.vi"("error in (no error)"=w664, "Delay and exposure table"=w660, "Camera controls"=w659, "Handle"=w663) -> ("error out"=w652:errorcluster, "Hout"=w651:u64)  [unwired: 1 out]
        n356 = call "SCGetImageSize.vi"("Handle"=w651, "error in (no error)"=w652) -> ("Hout"=w650:u64, "error out"=w634:errorcluster, "Horizontal size"=w639:i32, "Vertical size"=w638:i32)  [unwired: 2 out]
        n357 = Greater?(x=w639, y=w638) -> (0:w640:bool)
        n358 = Initialize Array(u16 0 ("dimension size"), w638, w639) -> (w632:u16[][])
        n359 = call "SCRun.vi"("error in (no error)"=w634, "Run mode"=0, "Handle"=w650) -> ("error out"=w647:errorcluster, "Hout"=w646:u64)  [unwired: 1 out]
        n360 = Select(t=w639, s=w640, f=w638) -> (s? t:f=w637:i32)
        n361 = property on="mainimg" class="IntGraph (strict)"("XScale.Maximum"=w637, "YScale.Maximum"=w637) -> ()  [unwired: 2 in, 2 out]
      }
      frame "bench" {
        n362 = Dequeue Element(queue=w675) -> ()  [unwired: 2 in, 4 out]
        n363 = call "SCStopCOC.vi"("error in (no error)"=w677, "Stop mode"=0, "Handle"=w685) -> ("error out"=w669:errorcluster, "Hout"=w670:u64)
        n364 = while {
          tunnel: w671 -> [w701]
          tunnel: w670 -> [w700]
          tunnel: w669 -> [w691]
          shift-right: [w697] -> _
          shift-left: _ -> [w696]
          tunnel: [w693] -> w668
          tunnel: [w692] -> w667
          tunnel: w666 -> [w688]
          tunnel: [w687] -> w665
          stop <- "stop" stop-if-true
          n365 = call "wait4trig.vi"("error in"=w691, "task/channels in"=w688) -> ("error out"=w690:errorcluster, "voltage out"=→"voltage out":dbl, "task out"=w687:refnum<k21>)  [unwired: 7 in]
          n366 = call "SCRun.vi"("error in (no error)"=w690, "Run mode"=4, "Handle"=w700) -> ("error out"=w702:errorcluster, "Hout"=w703:u64)  [unwired: 1 out]
          n367 = call <vilib>:"High Resolution Relative Seconds.vi"() -> ("relative seconds"=w697:dbl)
          n368 = call "grabimg.vi"("array in"=w701, "error in"=w702, "Hin"=w703) -> ("error out"=w692:errorcluster, "imgdata"=w699:i32[][], "Hout"=w693:u64)  [unwired: 6 in]
          n369 = To Double Precision Float(number=w699) -> (double precision float=→"sideimg 2":dbl[][])
          n370 = Subtract(x=w697, y=w696) -> (x-y=w694:dbl)
          "x/y" <- w694
          n371 = Reciprocal(x=w694) -> (1/x=→"1/x":dbl)
        }
        n372 = call "SCStopCOC.vi"("error in (no error)"=w667, "Stop mode"=0, "Handle"=w668) -> ("error out"=w672:errorcluster, "Hout"=w673:u64)
        n373 = call "SCRun.vi"("error in (no error)"=w672, "Run mode"=0, "Handle"=w673) -> ("error out"=w682:errorcluster, "Hout"=w681:u64)  [unwired: 1 out]
      }
      frame "release" {
        n374 = Dequeue Element(queue=w715) -> ()  [unwired: 2 in, 4 out]
        n375 = flat-sequence {
          tunnel: w713 -> [w717]
          tunnel: [w716] -> w710
          tunnel: [w719] -> w711
          tunnel: w710 -> [w719]
          frame #0 {
            n376 = call "SCCloseBoard.vi"("Handle"=w717) -> ("error out"=w716:errorcluster)  [unwired: 1 in, 2 out]
          }
          frame #1 {
            n377 = local write "cam_con?"(FALSE ("cam_con?")) -> ()
          }
        }
        n378 = call <vilib>:"DAQmx Clear Task.vi"("task in"=w706) -> ()  [unwired: 14 in, 1 out]
      }
      frame "close" {
        n379 = Release Queue(queue=w728) -> ()  [unwired: 2 in, 3 out]
      }
      frame "idle", Default {
        n380 = call "grabimg.vi"("array in"=w769, "error in"=w775, "Hin"=w776) -> ("error out"=w774:errorcluster, "imgdata"=w772:i32[][], "Hout"=w773:u64)  [unwired: 6 in]
        n381 = local read "lower threshold"() -> (w767:i32)
        n382 = case shown="False" "cam_dark?" {
          tunnel: w778 -> [_ w801]
          tunnel: [w798 w800] -> w768
          tunnel: w772 -> [w798 w799]
          frame False {
          }
          frame True {
            n383 = Subtract(x=w799, y=w801) -> (x-y=w800:dbl[][])
          }
        }
        n384 = call "filtr_b.vi"("threshold"=w767, "input array"=w768) -> ("output array"=w759:dbl[][])  [unwired: 9 in]
        n385 = call <vilib>:"High Resolution Relative Seconds.vi"() -> ("relative seconds"=w783:dbl)
        n386 = Subtract(x=w783, y=w782) -> (x-y=w781:dbl)
        n387 = Array Size(array=w759) -> (size(s)=w758:i32[])
        n388 = Reciprocal(x=w781) -> (1/x=→"cam_fps":dbl)
        n389 = Index Array(array=w758) -> (element #1=w753:i32, element #2=w752:i32)  [unwired: 2 in]
        n390 = Subtract(x=w744, y=w743) -> (x-y=w742:i32)
        n391 = Less Or Equal?(x="pics2avg", y=w742) -> (x <= y?=w765:bool)
        n392 = And(x="reset every n pics", y=w765) -> (x .and. y?=w763:bool)
        n393 = Not(x=w763) -> (.not. x?=w762:bool)
        n394 = call-poly <vilib>:"Ramp Pattern.vi"("start"=0.0, "end"=w753, "samples"=w753) -> ("Ramp Pattern"=w748:dbl[])  [unwired: 7 in, 1 out]
        n395 = call-poly <vilib>:"Ramp Pattern.vi"("start"=0.0, "end"=w752, "samples"=w752) -> ("Ramp Pattern"=w749:dbl[])  [unwired: 7 in, 1 out]
        n396 = property on="mainimg" class="IntGraph (strict)"() -> ("CrsrLis"=w741:T4)  [unwired: 2 in, 2 out]
        n397 = And(x="cam_liveavg", y=w762) -> (x .and. y?=w760:bool)
        n398 = case shown="False" w760 {
          tunnel: w759 -> [w788 w794]
          tunnel: [w788 w791] -> w736
          tunnel: w771 -> [_ w796]
          tunnel: w744 -> [w789 _]
          tunnel: [w789 w797] -> w770
          tunnel: w743 -> [_ w797]
          tunnel: w742 -> [_ w790]
          frame False {
          }
          frame True {
            n399 = Multiply(x=w796, y=w790) -> (x*y=w795:dbl[][])
            n400 = Increment(x=w790) -> (x+1=w792:i32)
            n401 = Add(x=w795, y=w794) -> (x+y=w793:dbl[][])
            n402 = Divide(x=w793, y=w792) -> (x/y=w791:dbl[][])
          }
        }
        "mainimg" <- w736
        n403 = Index Array(array=w741) -> (element #1=w739:T7, element #2=w740:T7)  [unwired: 2 in]
        n404 = Unbundle By Name(w739) -> ("Position.X"=w733:dbl, "Position.Y"=w735:dbl)
        n405 = Unbundle By Name(w740) -> ("Position.X"=w737:dbl, "Position.Y"=w738:dbl)
        n406 = Array Max & Min(array=w736) -> (max value=→"max":dbl)  [unwired: 3 out]
        n407 = Subtract(x=w738, y=w735) -> (x-y=w734:dbl)
        n408 = Subtract(x=w737, y=w733) -> (x-y=w732:dbl)
        n409 = Array Subset(array=w736, index (row)=w735, length (row)=w734) -> (w747:dbl[][])  [unwired: 2 in]
        n410 = Array Subset(array=w736, index (col)=w733, length (col)=w732) -> (w745:dbl[][])  [unwired: 2 in]
        n411 = Array Subset(array=w736, index (row)=w735, length (row)=w734, index (col)=w733, length (col)=w732) -> (w731:dbl[][])
        n412 = Transpose 2D Array(2D array=w747) -> (transposed array=w746:dbl[][])
        n413 = Add Array Elements(numeric array=w731) -> (sum=→"sum" →"Waveform Chart":dbl)
        n414 = for {
          tunnel: w745 -> [w785] mode=indexing
          tunnel: [w784] -> w755 mode=indexing
          n415 = Add Array Elements(numeric array=w785) -> (sum=w784:dbl)
        }
        n416 = for {
          tunnel: w746 -> [w787] mode=indexing
          tunnel: [w786] -> w754 mode=indexing
          n417 = Add Array Elements(numeric array=w787) -> (sum=w786:dbl)
        }
        n418 = Bundle("Ramp Pattern"=w749, w754) -> (→"G2 X":cluster{"Ramp Pattern":dbl[], dbl[]})  [unwired: 1 in]
        n419 = Bundle(w755, "Ramp Pattern"=w748) -> (→"G2 Y":cluster{dbl[], "Ramp Pattern":dbl[]})  [unwired: 1 in]
      }
      frame "dark" {
        n420 = Dequeue Element(queue=w816) -> ()  [unwired: 2 in, 4 out]
        n421 = Array Size(array=w813) -> (size(s)=w812:i32[])
        n422 = Index Array(array=w812) -> (element #1=w811:i32, element #2=w810:i32)  [unwired: 2 in]
        n423 = Initialize Array(0.0 ("element"), w811, w810) -> (w808:dbl[][])
        n424 = for {
          N: "dark avg" -> [_]
          tunnel: w818 -> [w826]
          tunnel: w817 -> [w825]
          tunnel: [w824] -> w815
          tunnel: w813 -> [w823]
          tunnel: [w822] -> w814
          shift-right: [w819] -> w806
          shift-left: w808 -> [w820]
          n425 = call "grabimg.vi"("array in"=w823, "error in"=w825, "Hin"=w826) -> ("error out"=w824:errorcluster, "imgdata"=w821:i32[][], "Hout"=w822:u64)  [unwired: 6 in]
          n426 = Add(x=w821, y=w820) -> (x+y=w819:dbl[][])
        }
        n427 = Divide(x=w806, y="dark avg") -> (x/y=w807:dbl[][])
      }
      frame "snap" {
        w836 = 0
        n428 = Dequeue Element(queue=w855) -> ()  [unwired: 2 in, 4 out]
        n429 = local read "cam_dark?"() -> (w854:bool)
        n430 = local read "averages"() -> (w849:i32)
        n431 = To Double Precision Float(number=w840) -> (double precision float=w839:dbl[][])
        n432 = Equal To 0?(x="aq.mode") -> (x = 0?=w842:bool)
        n433 = Get Date/Time In Seconds() -> (seconds since 1Jan1904=w845:timestamp)
        n434 = for {
          N: w849 -> [w875]
          shift-right: [w893] -> w850
          shift-left: w852 -> [w895]
          shift-right: [w880] -> w848
          shift-left: w851 -> [w894]
          tunnel: w854 -> [w891]
          tunnel: w853 -> [w890]
          tunnel: w840 -> [w889]
          tunnel: w845 -> [w885]
          tunnel: w842 -> [w868]
          shift-right: [w876] -> w830
          shift-left: w839 -> [w877]
          shift-right: [w861] -> w835
          shift-left: w839 -> [w867]
          shift-right: [w866] -> w837
          shift-left: w838 -> [w860]
          shift-right: [w857] -> _
          shift-left: w836 -> [w858]
          shift-right: [w856] -> _
          shift-left: w836 -> [w859]
          i -> [w864]
          stop <- "abort acq." stop-if-true
          n435 = call "grabimg.vi"("array in"=w889, "error in"=w894, "Hin"=w895) -> ("error out"=w880:errorcluster, "imgdata"=w892:i32[][], "Hout"=w893:u64)  [unwired: 6 in]
          n436 = local read "lower threshold"() -> (w871:i32)
          n437 = Increment(x=w864) -> (x+1=w873:i32)
          "acq. imgs" <- w873
          n438 = Get Date/Time In Seconds() -> (seconds since 1Jan1904=w888:timestamp)
          n439 = case shown="True" w891 {
            tunnel: w892 -> [w953 w956]
            tunnel: w890 -> [_ w955]
            tunnel: [w953 w954] -> w870
            frame False {
            }
            frame True {
              n440 = Subtract(x=w956, y=w955) -> (x-y=w954:dbl[][])
            }
          }
          n441 = Divide(x=w873, y=w875) -> (x/y=→"snap_prog":dbl)
          n442 = flat-sequence {
            tunnel: [w896] -> w866
            tunnel: [w900] -> w865
            tunnel: w863 -> [w899]
            tunnel: [w899] -> w862
            tunnel: [w898] -> _
            tunnel: w860 -> [w898]
            frame #0 {
              n443 = call-poly <vilib>:"DAQmx Read.vi"("task/channels in"=w898) -> ("task out"=w896:refnum<k21>, "data"=w897:dbl)  [unwired: 12 in, 1 out]
              "Voltage" <- w897
              n444 = Greater?(x=w897, y=2.5) -> (0:w900:bool)
            }
          }
          n445 = Subtract(x=w888, y=w885) -> (x-y=w887:dbl)
          n446 = call "filtr_b.vi"("threshold"=w871, "input array"=w870) -> ("output array"=w869:dbl[][])  [unwired: 9 in]
          n447 = Divide(x=w887, y=w864) -> (x/y=w883:dbl)
          n448 = Multiply(x=w883, y=w875) -> (x*y=w886:dbl)
          n449 = Reciprocal(x=w883) -> (1/x=w882:dbl)
          n450 = case shown="True" "count?" {
            tunnel: w869 -> [w942 w944]
            tunnel: "e-size" -> [_ w946]
            tunnel: w871 -> [_ w945]
            tunnel: [w942 w943] -> w863
            frame False {
            }
            frame True {
              n451 = Array Size(array=w944) -> (size(s)=w948:i32[])
              n452 = call "findr.vi"("thresh"=w945, "esize"=w946, "inp array"=w944) -> ("locs"=w947:i32[][])  [unwired: 8 in]
              n453 = Index Array(array=w948) -> (element #1=w950:i32, element #2=w949:i32)  [unwired: 2 in]
              n454 = call "drawe.vi"("Ysize"=w950, "Xsize"=w949, "pos array"=w947) -> ("img out"=w943:i32[][])  [unwired: 8 in]
            }
          }
          n455 = Add(x=w886, y=w885) -> (x+y=→"ETA":timestamp)
          n456 = local write "cam_fps"(w882) -> ()
          n457 = case shown="False" w865 {
            tunnel: w868 -> [w907 _]
            tunnel: w867 -> [w906 w921]
            tunnel: [w905 w921] -> w861
            tunnel: w862 -> [w904 _]
            tunnel: w859 -> [w903 w920]
            tunnel: [w902 w920] -> w856
            frame False {
              n458 = case shown="False" w907 {
                tunnel: w904 -> [w910 w918]
                tunnel: w903 -> [w909 w917]
                tunnel: w906 -> [w912 w916]
                tunnel: [w911 w914] -> w905
                tunnel: [w908 w913] -> w902
                frame False {
                  n459 = Add(x=w910, y=w912) -> (x+y=w911:dbl[][])
                  n460 = Increment(x=w909) -> (x+1=w908:i32)
                }
                frame True {
                  n461 = Multiply(x=w916, y=w917) -> (x*y=w919:dbl[][])
                  n462 = Increment(x=w917) -> (x+1=w913:i32)
                  n463 = Add(x=w918, y=w919) -> (x+y=w915:dbl[][])
                  n464 = Divide(x=w915, y=w913) -> (x/y=w914:dbl[][])
                }
              }
            }
            frame True {
            }
          }
          "Pics NL" <- w856
          n465 = case shown="True" w865 {
            tunnel: w877 -> [w923 w929]
            tunnel: [w923 w928] -> w876
            tunnel: w868 -> [_ w927]
            tunnel: w862 -> [_ w926]
            tunnel: w858 -> [w922 w925]
            tunnel: [w922 w924] -> w857
            frame False {
            }
            frame True {
              n466 = case shown="True" w927 {
                tunnel: w926 -> [w932 w940]
                tunnel: w925 -> [w931 w939]
                tunnel: w929 -> [w934 w938]
                tunnel: [w933 w936] -> w928
                tunnel: [w930 w935] -> w924
                frame False {
                  n467 = Add(x=w932, y=w934) -> (x+y=w933:dbl[][])
                  n468 = Increment(x=w931) -> (x+1=w930:i32)
                }
                frame True {
                  n469 = Multiply(x=w938, y=w939) -> (x*y=w941:dbl[][])
                  n470 = Increment(x=w939) -> (x+1=w935:i32)
                  n471 = Add(x=w940, y=w941) -> (x+y=w937:dbl[][])
                  n472 = Divide(x=w937, y=w935) -> (x/y=w936:dbl[][])
                }
              }
            }
          }
          "Pics L" <- w857
          n473 = local write "mainimg"(w869) -> ()
          n474 = Transpose 2D Array(2D array=w869) -> (transposed array=w881:dbl[][])
          n475 = for {
            tunnel: w881 -> [w952] mode=indexing
            tunnel: [w951] -> _ mode=indexing
            n476 = Add Array Elements(numeric array=w952) -> (sum=w951:dbl)
          }
          n477 = local write "sideimg"(w876) -> ()
          n478 = local write "sideimg 2"(w861) -> ()
        }
        n479 = Array Size(array=w830) -> (size(s)=w829:i32[])
        n480 = Index Array(array=w829) -> (element #1=w828:i32, element #2=w827:i32)  [unwired: 2 in]
        n481 = Reshape Array(w830, w828, w827, 2 ("dimension size")) -> (w831:dbl[][][])
        n482 = Insert Into Array(array=w831, index (dim 2)=1 ("disabled index (col)"), new element=w835) -> (w833:dbl[][][])  [unwired: 2 in]
        n483 = Enqueue Element(queue=w844, element=w833, error in (no error)=w848) -> (error out=w841:errorcluster)  [unwired: 1 in, 2 out]
      }
      frame "suspend" {
        n484 = Dequeue Element(queue=w965) -> ()  [unwired: 2 in, 4 out]
      }
    }
    "cam_error" <- w591
  }
  n485 = while {
    tunnel: w10 -> [w971]
    tunnel: w13 -> [w970]
    tunnel: w3 -> [w969]
    tunnel: w24 -> [w968]
    tunnel: w2 -> [w966]
    tunnel: w11 -> [w967]
    stop <- w972 stop-if-true
    n486 = event shown="[12] \"delscan_go 2\": Value Change" {
      selector: _ -> [_ _ _ _ _ _ _ _ _ _ _ _ _ _ _ _ _ _ _ _ _ _ _ _ _ _ _]
      dyn-events: _ -> [_ _ _ _ _ _ _ _ _ _ _ _ _ _ _ _ _ _ _ _ _ _ _ _ _ _ _]
      timeout: _ -> [_ _ _ _ _ _ _ _ _ _ _ _ _ _ _ _ _ _ _ _ _ _ _ _ _ _ _]
      tunnel: [_ TRUE _ _ _ _ _ _ _ _ _ _ _ _ _ _ _ _ _ _ _ _ _ _ _ _ _] -> w972
      tunnel: w971 -> [_ w985 w988 _ _ _ _ _ w1014 w1016 _ _ _ _ _ _ _ _ _ _ _ _ _ _ _ _ w1123]
      tunnel: w970 -> [_ w984 _ w992 _ _ _ _ _ _ _ _ _ _ _ _ _ w1049 _ w1061 _ _ _ _ _ _ _]
      tunnel: w969 -> [_ w983 _ _ w998 _ _ _ _ _ _ _ _ _ w1037 _ w1041 _ _ _ _ _ _ _ _ _ _]
      tunnel: w968 -> [_ w982 _ _ _ w1004 w1010 w1011 _ _ _ _ _ _ _ _ _ _ _ _ _ _ _ _ _ _ _]
      tunnel: w967 -> [_ w976 _ _ _ _ _ _ _ _ _ _ _ _ _ _ _ _ _ _ _ _ _ _ _ _ _]
      tunnel: w966 -> [_ w975 _ _ _ _ _ _ _ _ w1018 w1020 w1021 _ _ w1039 _ _ _ _ _ _ _ _ _ w1122 _]
      event Timeout {
        n487 = event-data() -> ()  [unwired: 1 in, 1 out]
        n488 = call-poly <vilib>:"Read Delimited Spreadsheet.vi"() -> ("all rows"=w973:string[][])  [unwired: 10 in, 5 out]
        n489 = local write "delay table [fs]"(w973) -> ()
      }
      event "main_close": Value Change {
        w974 = "close" ("element")
        w981 = "release" ("element")
        n490 = event-data() -> ()  [unwired: 1 in, 1 out]
        n491 = Release Queue(queue=w976) -> ()  [unwired: 2 in, 3 out]
        n492 = Enqueue Element(queue=w985, element=w981) -> (queue out=w980:refnum<queue>)  [unwired: 2 in, 2 out]
        n493 = Enqueue Element(queue=w984, element=w981) -> (queue out=w979:refnum<queue>)  [unwired: 2 in, 2 out]
        n494 = Enqueue Element(queue=w983, element=w981) -> (queue out=w978:refnum<queue>)  [unwired: 2 in, 2 out]
        n495 = Enqueue Element(queue=w982, element=w981) -> (queue out=w977:refnum<queue>)  [unwired: 2 in, 2 out]
        n496 = Enqueue Element(queue=w980, element=w974) -> ()  [unwired: 2 in, 3 out]
        n497 = Enqueue Element(queue=w979, element=w974) -> ()  [unwired: 2 in, 3 out]
        n498 = Enqueue Element(queue=w978, element=w974) -> ()  [unwired: 2 in, 3 out]
        n499 = Enqueue Element(queue=w977, element=w974) -> ()  [unwired: 2 in, 3 out]
        n500 = Enqueue Element(queue=w975, element=w974) -> ()  [unwired: 2 in, 3 out]
      }
      event "cam_release", "cam_init": Value Change {
        n501 = event-data() -> ()  [unwired: 1 in, 2 out]
        n502 = Select(t="init" ("name (unnamed)"), s="cam_init", f="release" ("name (unnamed)")) -> (s? t:f=w987:string)
        n503 = Enqueue Element(queue=w988, element=w987) -> ()  [unwired: 2 in, 3 out]
      }
      event "ESP_release", "ESP_init": Value Change {
        n504 = event-data() -> ()  [unwired: 1 in, 2 out]
        n505 = Select(t="init" ("name (unnamed)"), s="ESP_init", f="release" ("name (unnamed)")) -> (s? t:f=w996:string)
        n506 = Enqueue Element(queue=w992, element=w996) -> ()  [unwired: 2 in, 3 out]
      }
      event "manip_init", "manip_release": Value Change {
        n507 = event-data() -> ()  [unwired: 1 in, 2 out]
        n508 = Flush Queue(queue=w998) -> (queue out=w997:refnum<queue>)  [unwired: 1 in, 2 out]
        n509 = Select(t="init" ("name (unnamed)"), s="manip_init", f="release" ("name (unnamed)")) -> (s? t:f=w1000:string)
        n510 = Enqueue Element(queue=w997, element=w1000) -> ()  [unwired: 2 in, 3 out]
      }
      event "phoib_release", "phoib_init": Value Change {
        n511 = event-data() -> ()  [unwired: 1 in, 2 out]
        n512 = Flush Queue(queue=w1004) -> (queue out=w1003:refnum<queue>)  [unwired: 1 in, 2 out]
        n513 = Select(t="init" ("name (unnamed)"), s="phoib_init", f="release" ("name (unnamed)")) -> (s? t:f=w1006:string)
        n514 = Enqueue Element(queue=w1003, element=w1006) -> ()  [unwired: 2 in, 3 out]
      }
      event "phoib_standby": Value Change {
        n515 = event-data() -> ()  [unwired: 1 in, 2 out]
        n516 = Enqueue Element(queue=w1010, element="standby") -> ()  [unwired: 2 in, 3 out]
      }
      event "phoib_set": Value Change {
        n517 = event-data() -> ()  [unwired: 1 in, 2 out]
        n518 = Enqueue Element(queue=w1011, element="set") -> ()  [unwired: 2 in, 3 out]
      }
      event "cam_dark": Value Change {
        n519 = event-data() -> ()  [unwired: 1 in, 2 out]
        n520 = Enqueue Element(queue=w1014, element="dark") -> ()  [unwired: 2 in, 3 out]
      }
      event "ROI Left", "ROI Right", "ROI Top", "ROI Bottom", "exposure [ms]", "binning", "gain": Value Change {
        n521 = event-data() -> ()  [unwired: 1 in, 1 out]
        n522 = Enqueue Element(queue=w1016, element="set") -> ()  [unwired: 2 in, 3 out]
      }
      event "cam_saveimg": Value Change {
        n523 = event-data() -> ()  [unwired: 1 in, 1 out]
        n524 = Enqueue Element(queue=w1018, element="single") -> ()  [unwired: 2 in, 3 out]
      }
      event "delscan_go": Value Change {
        n525 = event-data() -> ()  [unwired: 1 in, 1 out]
        n526 = Enqueue Element(queue=w1020, element="GO") -> ()  [unwired: 2 in, 3 out]
      }
      event "delscan_go 2": Value Change {
        n527 = event-data() -> ()  [unwired: 1 in, 1 out]
        n528 = Enqueue Element(queue=w1021, element="delay_chop") -> ()  [unwired: 2 in, 3 out]
      }
      event "Move Abs": Value Change {
        n529 = event-data() -> ()  [unwired: 1 in, 1 out]
      }
      event "ManipRel +", "ManipRel -": Value Change {
        n530 = event-data() -> ()  [unwired: 1 in, 2 out]
        n531 = Negate(x="manip_deltas") -> (-x=w1025:dbl[])
        n532 = Select(t="manip_deltas", s="ManipRel +", f=w1025) -> (s? t:f=w1023:dbl[])
        n533 = Index Array(array=w1023) -> (element #1=w1029:dbl, element #2=w1030:dbl, element #3=w1031:dbl, element #4=w1032:dbl, element #5=w1033:dbl, element #6=w1034:dbl)  [unwired: 6 in]
        n534 = Format Into String(format string="%g_%g_%g_%g_%g_%g", w1029, w1030, w1031, w1032, w1033, w1034) -> (resulting string=w1036:string)  [unwired: 2 in, 1 out]
        n535 = Concatenate Strings("relative:" ("string"), w1036) -> (w1027:string)
        n536 = Enqueue Element(queue=w1037, element=w1027) -> ()  [unwired: 2 in, 3 out]
      }
      event "Optimize": Value Change {
        n537 = event-data() -> ()  [unwired: 1 in, 6 out]
        n538 = Enqueue Element(queue=w1039, element="manip") -> ()  [unwired: 2 in, 3 out]
      }
      event "stop manip": Value Change {
        n539 = event-data() -> ()  [unwired: 1 in, 1 out]
        n540 = Enqueue Element(queue=w1041, element="stop") -> ()  [unwired: 2 in, 3 out]
      }
      event "ESP_go": Value Change {
        w1043 = ":" ("string")
        n541 = event-data() -> ()  [unwired: 1 in, 1 out]
        n542 = local read "ESP Axis"() -> (w1042:i32)
        n543 = Number To Decimal String(number=w1042) -> (decimal integer string=w1045:string)  [unwired: 1 in]
        n544 = Number To Fractional String(number="ESP_dest") -> (F-format string=w1044:string)  [unwired: 3 in]
        n545 = Concatenate Strings("abs:" ("string"), w1045, w1043, w1044, w1043) -> (w1048:string)
        n546 = Enqueue Element(queue=w1049, element=w1048) -> ()  [unwired: 2 in, 3 out]
      }
      event "ESP_set_t0": Value Change {
        n547 = event-data() -> ()  [unwired: 1 in, 1 out]
        n548 = Current VI's Path() -> (path=w1055:path)
        n549 = Strip Path(path=w1055) -> (stripped path=w1051:path)  [unwired: 1 out]
        n550 = Strip Path(path=w1051) -> (stripped path=w1050:path)  [unwired: 1 out]
        n551 = local read "ESP_pos"() -> (w1053:dbl)
        "ESP_t0" <- w1053
        n552 = Number To Fractional String(number=w1053) -> (F-format string=w1052:string)  [unwired: 3 in]
        n553 = Build Path(base path=w1050, name or relative path="t0.txt") -> (appended path=w1054:path)
        n554 = Write to Text File(file (use dialog)=w1054, text=w1052) -> ()  [unwired: 2 in, 3 out]
      }
      event "ESP_+", "ESP_-": Value Change {
        n555 = event-data() -> ()  [unwired: 1 in, 6 out]
        n556 = Negate(x="ESP_delta") -> (-x=w1064:dbl)
        n557 = Select(t="ESP_delta", s="ESP_+", f=w1064) -> (s? t:f=w1062:dbl)
        n558 = Number To Decimal String(number="ESP Axis") -> (decimal integer string=w1059:string)  [unwired: 1 in]
        n559 = Number To Fractional String(number=w1062) -> (F-format string=w1057:string)  [unwired: 3 in]
        n560 = Concatenate Strings("rel:" ("string"), w1059, ":" ("string"), w1057) -> (w1067:string)
        n561 = Enqueue Element(queue=w1061, element=w1067) -> ()  [unwired: 2 in, 3 out]
      }
      event "ESP_dest": Value Change {
        n562 = event-data() -> ()  [unwired: 1 in, 6 out]
        n563 = local read "ESP_dest"() -> (w1071:dbl)
        n564 = local read "ESP_t0"() -> (w1070:dbl)
        n565 = call "mm2time.vi"("fs?"=TRUE ("fs[1]/ps[0]"), "Offset (mm)"=w1070, "distance (mm)"=w1071) -> ("time in fs/ps seconds"=w1068:dbl)
        n566 = local write "ESP_dest_t"(w1068) -> ()
      }
      event "ESP_dest_t": Value Change {
        n567 = event-data() -> ()  [unwired: 1 in, 1 out]
        n568 = local read "ESP_t0"() -> (w1074:dbl)
        n569 = call "time2mm.vi"("fs[1]/ps[0]"=TRUE, "Offset (mm)"=w1074, "time"="ESP_dest_t") -> ("position (mm)"=w1072:dbl)
        n570 = local write "ESP_dest"(w1072) -> ()
      }
      event "load delay table": Value Change {
        n571 = event-data() -> ()  [unwired: 1 in, 6 out]
        n572 = call-poly <vilib>:"Read Delimited Spreadsheet.vi"() -> ("all rows"=w1077:string[][])  [unwired: 10 in, 5 out]
        n573 = local read "binning"() -> (w1084:u16)
        n574 = local write "delay table [fs]"(w1077) -> ()
        n575 = local read "delscan_iters"() -> (w1078:u32)
        n576 = local read "time / step"() -> (w1087:dbl)
        n577 = Array Size(array=w1077) -> (size(s)=w1088:i32[])
        n578 = Index Array(array=dbl[] [8.79, 2.2, 0.553, 0.138], index=w1084) -> (element=w1082:dbl)
        n579 = Index Array(array=w1088) -> (element #1=w1076:i32)  [unwired: 2 in, 1 out]
        n580 = Multiply(x=w1078, y=w1076) -> (x*y=w1081:u32)
        n581 = Multiply(x=w1076, y=w1082) -> (x*y=w1083:dbl)
        n582 = Multiply(x=w1081, y=w1087) -> (x*y=w1086:dbl)
        n583 = Increment(x=w1081) -> (x+1=w1080:u32)
        n584 = Multiply(x=w1080, y=w1082) -> (x*y=w1079:dbl)
        n585 = local write "delaypoints"(w1076) -> ()
        n586 = local write "total steps"(w1081) -> ()
        n587 = local write "duration [HH:MM:SS]"(w1086) -> ()
        n588 = local write "RAM [MB]"(w1083) -> ()
        n589 = local write "disk [MB]"(w1079) -> ()
      }
      event "delay table [fs]", "delscan_iters": Value Change {
        n590 = event-data() -> ()  [unwired: 1 in, 6 out]
        n591 = local read "binning"() -> (w1097:u16)
        n592 = local read "delay table [fs]"() -> (w1101:string[][])
        n593 = local read "delscan_iters"() -> (w1091:u32)
        n594 = local read "time / step"() -> (w1099:dbl)
        n595 = Array Size(array=w1101) -> (size(s)=w1100:i32[])
        n596 = Index Array(array=dbl[] [8.79, 2.2, 0.553, 0.138], index=w1097) -> (element=w1095:dbl)
        n597 = Index Array(array=w1100) -> (element #1=w1089:i32)  [unwired: 2 in, 1 out]
        n598 = Multiply(x=w1091, y=w1089) -> (x*y=w1094:u32)
        n599 = Multiply(x=w1089, y=w1095) -> (x*y=w1096:dbl)
        n600 = Multiply(x=w1094, y=w1099) -> (x*y=w1098:dbl)
        n601 = Increment(x=w1094) -> (x+1=w1093:u32)
        n602 = Multiply(x=w1093, y=w1095) -> (x*y=w1092:dbl)
        n603 = local write "delaypoints"(w1089) -> ()
        n604 = local write "total steps"(w1094) -> ()
        n605 = local write "duration [HH:MM:SS]"(w1098) -> ()
        n606 = local write "RAM [MB]"(w1096) -> ()
        n607 = local write "disk [MB]"(w1092) -> ()
      }
      event "generate delay table": Value Change {
        n608 = event-data() -> ()  [unwired: 1 in, 1 out]
        n609 = call "getdelaypoints.vi"("delscan_stepsize"="delscan_stepsize", "delscan_end"="delscan_end", "delscan_start"="delscan_start") -> ("delaypoints"=w1117:dbl[])
        n610 = Number To Fractional String(number=w1117) -> (F-format string=w1116:string[])  [unwired: 3 in]
        n611 = Build Array(w1116) -> (w1115:string[][])
        n612 = Transpose 2D Array(2D array=w1115) -> (transposed array=w1102:string[][])
        n613 = local write "delay table [fs]"(w1102) -> ()
        n614 = local read "binning"() -> (w1111:u16)
        n615 = local read "delscan_iters"() -> (w1105:u32)
        n616 = local read "time / step"() -> (w1113:dbl)
        n617 = Array Size(array=w1102) -> (size(s)=w1114:i32[])
        n618 = Index Array(array=dbl[] [8.79, 2.2, 0.553, 0.138], index=w1111) -> (element=w1109:dbl)
        n619 = Index Array(array=w1114) -> (element #1=w1103:i32)  [unwired: 2 in, 1 out]
        n620 = Multiply(x=w1105, y=w1103) -> (x*y=w1108:u32)
        n621 = Multiply(x=w1103, y=w1109) -> (x*y=w1110:dbl)
        n622 = Multiply(x=w1108, y=w1113) -> (x*y=w1112:dbl)
        n623 = Increment(x=w1108) -> (x+1=w1107:u32)
        n624 = Multiply(x=w1107, y=w1109) -> (x*y=w1106:dbl)
        n625 = local write "delaypoints"(w1103) -> ()
        n626 = local write "total steps"(w1108) -> ()
        n627 = local write "duration [HH:MM:SS]"(w1112) -> ()
        n628 = local write "RAM [MB]"(w1110) -> ()
        n629 = local write "disk [MB]"(w1106) -> ()
      }
      event "mainimg": Cursor Release {
        n630 = event-data() -> ()  [unwired: 1 in, 1 out]
        n631 = Enqueue Element(queue=w1122, element="refresh") -> ()  [unwired: 2 in, 3 out]
      }
      event "dev_bench": Value Change {
        n632 = event-data() -> ()  [unwired: 1 in, 2 out]
        n633 = Enqueue Element(queue=w1123, element="bench") -> ()  [unwired: 2 in, 3 out]
      }
    }
  }
  n634 = while {
    tunnel: w13 -> [w1133]
    shift-right: [w1131] -> _
    shift-left: _ -> [w1129]
    shift-right: [w1130] -> _
    shift-left: _ -> [w1128]
    shift-right: [w1126] -> _
    shift-left: 0 -> [w1127]
    tunnel: w2 -> [w1125]
    stop <- w1132 stop-if-true
    # "ESP"
    n635 = Preview Queue Element(queue=w1133, timeout in ms (-1)=w1127) -> (queue out=w1136:refnum<queue>, element=w1137:string)  [unwired: 1 in, 2 out]
    n636 = Match Pattern(string=w1137, regular expression=":") -> (before substring=w1135:string, after substring=w1134:string)  [unwired: 1 in, 2 out]
    n637 = case shown="\"init\"" w1135 {
      tunnel: w1136 -> [_ w1148 w1166 w1200 w1201 w1208 w1213]
      tunnel: w1134 -> [_ w1153 w1173 _ _ _ _]
      tunnel: [_ _ _ _ _ TRUE _] -> w1132
      tunnel: [w1140 w1155 w1167 w1198 refnum<visa-resource-name> refnum ("VISA resource name out") w1205 w1212] -> w1131
      tunnel: [w1139 w1156 w1165 w1197 w1203 w1206 w1211] -> w1130
      tunnel: w1129 -> [w1144 w1158 w1171 w1198 w1204 w1205 _]
      tunnel: w1128 -> [w1143 w1157 w1172 w1197 _ w1206 _]
      tunnel: [_ _ _ -1 _ _ _] -> w1126
      tunnel: w1125 -> [_ _ w1164 _ _ _ _]
      frame "idle", Default {
        n638 = local read "ESP Axis"() -> (w1141:i32)
        n639 = local read "ESP_t0"() -> (w1147:dbl)
        n640 = call "Read Actual Position.vi"("error in (no error)"=w1143, "Axis (1)"=w1141, "VISA resource name"=w1144) -> ("error out"=w1139:errorcluster, "Position (units)"=w1142:dbl, "VISA resource name out"=w1140:refnum<visa-resource-name>)  [unwired: 2 in]
        "ESP_pos" <- w1142
        n641 = call "mm2time.vi"("fs?"=TRUE, "Offset (mm)"=w1147, "distance (mm)"=w1142) -> ("time in fs/ps seconds"=→"ESP_delay":dbl)
      }
      frame "rel" {
        n642 = Match Pattern(string=w1153, regular expression=":") -> (before substring=w1152:string, after substring=w1151:string)  [unwired: 1 in, 2 out]
        n643 = Dequeue Element(queue=w1148) -> ()  [unwired: 2 in, 4 out]
        n644 = Decimal String To Number(string=w1152) -> (number=w1150:i32)  [unwired: 2 in, 1 out]
        n645 = Fract/Exp String To Number(string=w1151) -> (number=w1149:dbl)  [unwired: 3 in, 1 out]
        n646 = call "Move Relative.vi"("error in (no error)"=w1157, "Position (0 units)"=w1149, "Axis (1)"=w1150, "VISA resource name"=w1158) -> ("error out"=w1156:errorcluster, "VISA resource name out"=w1155:refnum<visa-resource-name>)  [unwired: 2 in]
      }
      frame "abs" {
        n647 = Dequeue Element(queue=w1166) -> ()  [unwired: 2 in, 4 out]
        n648 = Match Pattern(string=w1173, regular expression=":") -> (before substring=w1174:string, after substring=w1162:string)  [unwired: 1 in, 2 out]
        n649 = Match Pattern(string=w1162, regular expression=":") -> (before substring=w1161:string, after substring=w1160:string)  [unwired: 1 in, 2 out]
        n650 = Decimal String To Number(string=w1174) -> (number=w1170:i32)  [unwired: 2 in, 1 out]
        n651 = Fract/Exp String To Number(string=w1161) -> (number=w1159:dbl)  [unwired: 3 in, 1 out]
        n652 = call "Move Absolute.vi"("error in (no error)"=w1172, "Position (0 units)"=w1159, "Axis (1)"=w1170, "VISA resource name"=w1171) -> ("error out"=w1168:errorcluster, "VISA resource name out"=w1169:refnum<visa-resource-name>)  [unwired: 2 in]
        n653 = case shown="\"wait\"" w1160 {
          tunnel: w1170 -> [_ w1182]
          tunnel: w1169 -> [w1177 w1187]
          tunnel: w1168 -> [w1176 w1186]
          tunnel: [w1177 w1179] -> w1167
          tunnel: [w1176 w1185] -> w1165
          tunnel: w1164 -> [_ w1184]
          frame "", Default {
          }
          frame "wait" {
            n654 = while {
              tunnel: w1182 -> [w1196]
              shift-right: [w1193] -> w1181
              shift-left: w1187 -> [w1195]
              shift-right: [w1192] -> w1180
              shift-left: w1186 -> [w1194]
              stop <- w1191 stop-if-true
              n655 = call "Get Axis Motion Status.vi"("error in (no error)"=w1194, "Axis (1)"=w1196, "VISA resource name"=w1195) -> ("error out"=w1192:errorcluster, "Motion Done"=w1191:bool, "VISA resource name out"=w1193:refnum<visa-resource-name>)  [unwired: 2 in]
            }
            n656 = flat-sequence {
              tunnel: w1181 -> [w1190]
              tunnel: w1180 -> [w1189]
              tunnel: [w1190] -> w1179
              tunnel: [w1189] -> w1178
              frame #0 {
                n657 = Wait (ms)(milliseconds to wait=u32 1000) -> ()  [unwired: 1 out]
              }
            }
            n658 = Enqueue Element(queue=w1184, element="done", error in (no error)=w1178) -> (error out=w1185:errorcluster)  [unwired: 1 in, 2 out]
          }
        }
      }
      frame "suspend" {
        n659 = Dequeue Element(queue=w1200) -> ()  [unwired: 2 in, 4 out]
      }
      frame "release" {
        n660 = Dequeue Element(queue=w1201) -> ()  [unwired: 2 in, 4 out]
        n661 = call "Close.vi"("VISA resource name"=w1204) -> ("error out"=w1203:errorcluster)  [unwired: 10 in]
      }
      frame "close" {
        n662 = Release Queue(queue=w1208) -> ()  [unwired: 2 in, 3 out]
      }
      frame "init" {
        n663 = Dequeue Element(queue=w1213) -> ()  [unwired: 2 in, 4 out]
        n664 = flat-sequence {
          tunnel: [w1216] -> w1210
          tunnel: [w1215] -> w1209
          tunnel: [w1220] -> w1211
          tunnel: [w1221] -> w1212
          tunnel: w1210 -> [w1221]
          tunnel: w1209 -> [w1220]
          frame #0 {
            n665 = local write "ESP_con?"(FALSE ("ESP_con?")) -> ()
          }
          frame #1 {
            n666 = call "Initialize.vi"("VISA resource name"="ESP301 VISA", "Serial Link (RS232)"=enum16{"RS232", "USB"}."USB") -> ("VISA resource name out"=w1216:refnum<visa-resource-name>, "error out"=w1215:errorcluster)  [unwired: 7 in]
          }
          frame #2 {
            n667 = local write "ESP_con?"(TRUE ("ESP_con?")) -> ()
          }
        }
      }
    }
    "error out" <- w1130
  }
  n668 = while {
    tunnel: w3 -> [w1230]
    shift-right: [w1228] -> _
    shift-left: _ -> [w1226]
    shift-right: [w1227] -> _
    shift-left: _ -> [w1225]
    shift-right: [w1223] -> _
    shift-left: 0 -> [w1224]
    tunnel: w2 -> [w1222]
    stop <- w1229 stop-if-true
    # "manip"
    n669 = Preview Queue Element(queue=w1230, timeout in ms (-1)=w1224) -> (queue out=w1233:refnum<queue>, element=w1234:string)  [unwired: 1 in, 2 out]
    n670 = Match Pattern(string=w1234, regular expression=":") -> (before substring=w1232:string, after substring=w1231:string)  [unwired: 1 in, 2 out]
    n671 = case shown="\"init\"" w1232 {
      tunnel: w1233 -> [_ w1246 w1273 w1300 w1304 w1313 w1318]
      tunnel: w1231 -> [_ _ w1260 _ _ _ _]
      tunnel: [_ _ _ _ _ TRUE _] -> w1229
      tunnel: [w1240 w1248 w1252 w1302 refnum<k5> refnum ("gateway_connection out") w1311 w1317] -> w1228
      tunnel: [w1239 w1247 w1254 w1301 w1306 w1310 w1316] -> w1227
      tunnel: w1226 -> [w1242 w1250 w1276 w1302 w1308 w1311 _]
      tunnel: w1225 -> [w1241 w1249 w1275 w1301 _ w1310 _]
      tunnel: [_ _ _ -1 _ _ _] -> w1223
      tunnel: w1222 -> [_ _ w1251 _ _ _ _]
      frame "idle", Default {
        n672 = call "sp_manip_get_axis_status.vi"("error in"=w1241, "gateway_connection"=w1242) -> ("error out"=w1239:errorcluster, "axis_out"=w1238:T8, "gateway_connection out"=w1240:refnum<k5>)  [unwired: 5 in, 2 out]
        n673 = for {
          tunnel: w1238 -> [w1245] mode=indexing
          tunnel: [w1244] -> w1237 mode=indexing
          tunnel: [w1243] -> w1236 mode=indexing
          n674 = Unbundle By Name(w1245) -> ("Axis_Position"=w1244:dbl, "moving"=w1243:bool)
        }
        "moving?" <- w1236
        n675 = local write "pos"(w1237) -> ()
      }
      frame "stop" {
        n676 = Dequeue Element(queue=w1246) -> ()  [unwired: 2 in, 4 out]
        n677 = call "sp_manip_abort.vi"("error in"=w1249, "gateway_connection"=w1250) -> ("error out"=w1247:errorcluster, "gateway_connection out"=w1248:refnum<k5>)  [unwired: 6 in, 2 out]
      }
      frame "relative" {
        n678 = Dequeue Element(queue=w1273) -> ()  [unwired: 2 in, 4 out]
        n679 = Match Pattern(string=w1260, regular expression=":") -> (before substring=w1259:string, after substring=w1258:string)  [unwired: 1 in, 2 out]
        n680 = Equal?(x=w1258, y="wait") -> (x = y?=w1256:bool)
        n681 = call "sp_manip_get_axis_status.vi"("error in"=w1275, "gateway_connection"=w1276) -> ("error out"=w1278:errorcluster, "axis_out"=w1265:T8, "gateway_connection out"=w1277:refnum<k5>)  [unwired: 5 in, 2 out]
        n682 = Scan From String(format string="%g_%g_%g_%g_%g_%g", input string=w1259) -> (output 1=w1272:dbl, output 2=w1271:dbl, output 3=w1270:dbl, output 4=w1269:dbl, output 5=w1268:dbl, output 6=w1267:dbl)  [unwired: 8 in, 3 out]
        n683 = for {
          tunnel: w1265 -> [w1299] mode=indexing
          tunnel: [w1298] -> w1263 mode=indexing
          tunnel: [w1297] -> w1264 mode=indexing
          n684 = Unbundle By Name(w1299) -> ("Axis_Name"=w1298:string, "Axis_Position"=w1297:dbl)
        }
        n685 = Build Array(w1272, w1271, w1270, w1269, w1268, w1267) -> (w1266:dbl[])
        n686 = Add(x=w1264, y=w1266) -> (x+y=w1262:dbl[])
        n687 = call "sp_manip_start_move.vi"("error in"=w1278, "target positions"=w1262, "axis names"=w1263, "gateway_connection"=w1277) -> ("error out"=w1255:errorcluster, "gateway_connection out"=w1253:refnum<k5>)  [unwired: 4 in, 2 out]
        n688 = case shown="True" w1256 {
          tunnel: w1255 -> [w1279 w1286]
          tunnel: [w1279 w1282] -> w1254
          tunnel: w1253 -> [w1280 w1287]
          tunnel: [w1280 w1285] -> w1252
          tunnel: w1251 -> [_ w1281]
          frame False {
          }
          frame True {
            n689 = while {
              tunnel: w1287 -> [w1291]
              tunnel: w1286 -> [w1290]
              tunnel: [w1289] -> w1285
              tunnel: [w1288] -> w1283
              stop <- w1292 continue-if-true
              n690 = call "sp_manip_get_axis_status.vi"("error in"=w1290, "gateway_connection"=w1291) -> ("error out"=w1288:errorcluster, "axis_out"=w1294:T8, "gateway_connection out"=w1289:refnum<k5>)  [unwired: 5 in, 2 out]
              n691 = for {
                tunnel: w1294 -> [w1296] mode=indexing
                tunnel: [w1295] -> w1293 mode=indexing
                n692 = Unbundle By Name(w1296) -> ("moving"=w1295:bool)
              }
              n693 = Or Array Elements(Boolean array=w1293) -> (logical OR=w1292:bool)
            }
            n694 = Enqueue Element(queue=w1281, element="done", error in (no error)=w1283) -> (error out=w1282:errorcluster)  [unwired: 1 in, 2 out]
          }
        }
      }
      frame "suspend" {
        n695 = Dequeue Element(queue=w1300) -> ()  [unwired: 2 in, 4 out]
      }
      frame "release" {
        n696 = Dequeue Element(queue=w1304) -> ()  [unwired: 2 in, 4 out]
        n697 = call "sp_manip_disconnect.vi"("gateway_connection"=w1308) -> ("error out"=w1307:errorcluster, "gateway_connection_out"=w1309:refnum<k5>)  [unwired: 7 in, 2 out]
        n698 = call "tcp_gateway_close_connection.vi"("error in"=w1307, "server_connection"=w1309) -> ("error out"=w1306:errorcluster)  [unwired: 5 in]
      }
      frame "close" {
        n699 = Release Queue(queue=w1313) -> ()  [unwired: 2 in, 3 out]
      }
      frame "init" {
        n700 = Dequeue Element(queue=w1318) -> ()  [unwired: 2 in, 4 out]
        n701 = flat-sequence {
          tunnel: [w1321] -> w1315
          tunnel: [w1320] -> w1314
          tunnel: [w1331] -> w1316
          tunnel: [w1332] -> w1317
          tunnel: w1315 -> [w1332]
          tunnel: w1314 -> [w1331]
          frame #0 {
            n702 = local write "manip_con?"(FALSE ("manip_con?")) -> ()
          }
          frame #1 {
            n703 = call "tcp_gateway_open_connection.vi"() -> ("gateway_connection"=w1324:refnum<k5>, "error out"=w1323:errorcluster)  [unwired: 5 in, 3 out]
            n704 = call "sp_manip_connect.vi"("error in"=w1323, "gateway_connection"=w1324) -> ("error out"=w1320:errorcluster, "axis_out"=w1322:T8, "gateway_connection out"=w1321:refnum<k5>)  [unwired: 5 in, 2 out]
            n705 = for {
              tunnel: w1322 -> [w1329] mode=indexing
              tunnel: [w1328] -> w1325 mode=indexing
              tunnel: [w1327] -> w1326 mode=indexing
              n706 = Unbundle By Name(w1329) -> ("Axis_Name"=w1328:string, "Axis_Position"=w1327:dbl)
            }
            "axis" <- w1325
            "pos" <- w1326
            n707 = local write "dest"(w1326) -> ()
          }
          frame #2 {
            n708 = local write "manip_con?"(TRUE ("manip_con?")) -> ()
          }
        }
      }
    }
    "error out 2" <- w1227
  }
  n709 = while {
    tunnel: w24 -> [w1343]
    shift-right: [w1340] -> _
    shift-left: 0 -> [w1341]
    shift-right: [w1339] -> _
    shift-left: _ -> [w1338]
    shift-right: [w1337] -> _
    shift-left: _ -> [w1336]
    shift-right: [w1335] -> _
    shift-left: u32 0 ("pHandle") -> [w1334]
    tunnel: string[] ["Kinetic Energy", "Pass Energy", "Coil Current", "Work Function", "Detector Voltage", "Screen Voltage", "Conversion Voltage", "Focus Displacement 1", "Focus Displacement 2"] -> [w1333]
    stop <- w1342 stop-if-true
    # "phoib"
    n710 = Preview Queue Element(queue=w1343, timeout in ms (-1)=w1341) -> (queue out=w1346:refnum<queue>, element=w1347:string)  [unwired: 1 in, 2 out]
    n711 = Match Pattern(string=w1347, regular expression=":") -> (before substring=w1345:string, after substring=w1344:string)  [unwired: 1 in, 2 out]
    n712 = case shown="\"standby\"" w1345 {
      tunnel: w1346 -> [_ w1400 w1416 w1432 w1446 w1450 w1456]
      tunnel: w1344 -> [_ _ _ _ _ _ _]
      tunnel: [_ _ _ _ TRUE _ _] -> w1342
      tunnel: [_ _ _ _ _ -1 _] -> w1340
      tunnel: [w1357 w1402 w1419 w1430 w1444 w1449 w1453] -> w1339
      tunnel: w1338 -> [w1368 w1391 w1421 w1431 w1444 w1449 _]
      tunnel: [w1356 w1401 w1418 w1429 w1442 w1447 w1452] -> w1337
      tunnel: w1336 -> [w1366 w1390 w1420 _ w1442 w1447 _]
      tunnel: [w1354 w1388 w1417 w1428 w1443 w1448 w1455] -> w1335
      tunnel: w1334 -> [w1354 w1388 w1417 w1427 w1443 w1448 _]
      tunnel: w1333 -> [w1355 w1381 _ _ _ _ _]
      frame "idle", Default {
        n713 = call "SL2_AD_DLL_Phoibos_GetDeviceState.vi"("dll_path"=w1368, "pHandle_in"=w1354, "dev_type"=DEF_dev_type."devA (analyzer)", "error in"=w1366) -> ("path out"=w1353:path, "state"=→"state":T3, "error out"=w1352:errorcluster)  [unwired: 2 in]
        n714 = for {
          tunnel: w1354 -> [w1375]
          tunnel: w1355 -> [w1373] mode=indexing
          tunnel: [w1372] -> w1365 mode=indexing
          tunnel: [w1371] -> w1357
          shift-right: [w1370] -> w1356
          shift-left: w1352 -> [w1374]
          tunnel: w1353 -> [w1369]
          n715 = call "SL2_AD_DLL_Phoibos_GetVoltage.vi"("error in"=w1374, "voltage_name"=w1373, "pHandle"=w1375, "dll path in"=w1369) -> ("error out"=w1370:errorcluster, "value"=w1372:dbl, "dll path out"=w1371:path)  [unwired: 3 in]
        }
        n716 = Index Array(array=w1365) -> (element #1=→"phoib_I_1":dbl, element #2=→"phoib_I_2":dbl, element #3=→"phoib_I_3":dbl, element #4=→"phoib_I_4":dbl, element #5=→"phoib_I_5":dbl, element #6=→"phoib_I_6":dbl, element #7=→"phoib_I_7":dbl, element #8=→"phoib_I_8":dbl, element #9=→"phoib_I_9":dbl)  [unwired: 9 in]
      }
      frame "set" {
        n717 = Dequeue Element(queue=w1400) -> ()  [unwired: 2 in, 4 out]
        n718 = Multiply(x="VoltageRange", y=13) -> (x*y=w1397:i32)
        n719 = Add(x="Mode", y=w1397) -> (x+y=w1394:i32)
        n720 = Index Array(array=u32[] [251749632, 251749633, 251749634, 251749635, 251749636, 251749637, 251749638, 251749639, 251749640, 251749641, 251749642, 251749643, 251749644, 251749645, 251749646, 251749647, 251749648, 251749649, 251749650, 251749651, 251749652, 251749653, 251749654, 251749655, 251749656, 251749657, 251749658, 251749659, 251749660, 251749661, 251749662, 251749663, 251749664, 251749665, 251749666, 251749667, 251749668, 251749669, 251749670, 251749671, 251749672, 251749673, 251749674, 251749675, 251749676, 251749677, 251749678, 251749679, 251749680, 251749681, 251749682, 251749683, 251749684, 251749685, 251749686, 251749687, 251749688, 251749689, 251749690, 251749691, 251749692, 251749693, 251749694, 251749695, 251749696] ("modeIDs"), index=w1394) -> (element=w1392:u32)
        n721 = Build Array("phoib_I_1s", "phoib_I_2s", "phoib_I_3s", "phoib_I_4s", "phoib_I_5s", "phoib_I_6s", "phoib_I_7s", "phoib_I_8s", "phoib_I_9s") -> (w1380:dbl[])
        n722 = call "SL2_AD_DLL_Phoibos_SetDeviceMode.vi"("pHandle"=w1388, "error in"=w1390, "value"=w1392, "dev_type"=DEF_dev_type."devA (analyzer)", "dll path in"=w1391) -> ("error out"=w1379:errorcluster, "dll path out"=w1389:path)  [unwired: 4 in]
        n723 = for {
          tunnel: w1388 -> [w1408]
          shift-right: [w1415] -> w1402
          shift-left: w1389 -> [w1412]
          tunnel: w1381 -> [w1407] mode=indexing
          tunnel: w1380 -> [w1406] mode=indexing
          shift-right: [w1414] -> w1401
          shift-left: w1379 -> [w1410]
          n724 = call "SL2_AD_DLL_Phoibos_GetVoltageRange.vi"("error in"=w1410, "voltage_name"=w1407, "pHandle"=w1408, "dll path in"=w1412) -> ("error out"=w1409:errorcluster, "min"=w1404:dbl, "max"=w1405:dbl, "dll path out"=w1411:path)  [unwired: 2 in]
          n725 = In Range and Coerce(upper limit=w1405, x=w1406, lower limit=w1404) -> (coerced(x)=w1403:dbl)  [unwired: 1 out]
          n726 = call "SL2_AD_DLL_Phoibos_SetVoltage.vi"("commit"=TRUE, "pHandle"=w1408, "error in"=w1409, "value"=w1403, "voltageName"=w1407, "dll path in"=w1411) -> ("error out"=w1414:errorcluster, "dll path out"=w1415:path)  [unwired: 3 in]
        }
      }
      frame "standby" {
        w1422 = T3 0 items=["Off"=-1, "Standby"=0, "On"=1] ("state")
        n727 = Dequeue Element(queue=w1416) -> ()  [unwired: 2 in, 4 out]
        n728 = call "SL2_AD_DLL_Phoibos_SetDeviceState.vi"("pHandle_in"=w1417, "error in"=w1420, "state"=w1422, "dev_type"=DEF_dev_type."devA (analyzer)", "dll_path"=w1421) -> ("error out"=w1418:errorcluster, "path out"=w1419:path)  [unwired: 2 in]
      }
      frame "release" {
        n729 = Dequeue Element(queue=w1432) -> ()  [unwired: 2 in, 4 out]
        n730 = flat-sequence {
          tunnel: w1431 -> [w1433]
          tunnel: w1427 -> [w1434]
          tunnel: [w1437] -> w1426
          tunnel: [w1436] -> w1425
          tunnel: [u32 0] -> w1424
          tunnel: [w1439] -> w1428
          tunnel: [w1440] -> w1429
          tunnel: [w1441] -> w1430
          tunnel: w1426 -> [w1441]
          tunnel: w1425 -> [w1440]
          tunnel: w1424 -> [w1439]
          frame #0 {
            n731 = call "SL2_AD_DLL_Phoibos_Shutdown.vi"("pHandle"=w1434, "dll path in"=w1433) -> ("error out"=w1436:errorcluster, "dll path out"=w1437:path)  [unwired: 4 in]
          }
          frame #1 {
            n732 = local write "phoib_con?"(FALSE ("phoib_con?")) -> ()
          }
        }
      }
      frame "close" {
        n733 = Release Queue(queue=w1446) -> ()  [unwired: 2 in, 3 out]
      }
      frame "suspend" {
        n734 = Dequeue Element(queue=w1450) -> ()  [unwired: 2 in, 4 out]
      }
      frame "init" {
        n735 = Dequeue Element(queue=w1456) -> ()  [unwired: 2 in, 4 out]
        n736 = flat-sequence {
          tunnel: [w1463] -> w1454
          tunnel: [w1459] -> w1453
          tunnel: [w1458] -> w1452
          tunnel: [w1471] -> w1455
          tunnel: w1454 -> [w1471]
          frame #0 {
            n737 = local write "phoib_con?"(FALSE ("phoib_con?")) -> ()
          }
          frame #1 {
            w1462 = DEF_dev_type."devA (analyzer)" ("dev_type")
            n738 = call "GetSL2AD_VI_dllPath.vi"() -> ("error"=w1466:errorcluster, "Path"=w1467:path)  [unwired: 9 in, 1 out]
            n739 = call "SL2_AD_DLL_List_Devices.vi"("error in"=w1466, "dev_type"=w1462, "dll path in"=w1467) -> ("error out"=w1460:errorcluster, "devices"=w1469:string[], "dll path out"=w1461:path)  [unwired: 2 in]
            n740 = Index Array(array=w1469) -> (element=w1468:string)  [unwired: 1 in]
            n741 = call "SL2_AD_DLL_Phoibos_Initialize.vi"("error in"=w1460, "analyzerId"=w1468, "dll_path"=w1461) -> ("error out"=w1464:errorcluster, "pHandle"=w1463:u32, "path out"=w1465:path)  [unwired: 2 in]
            n742 = call "SL2_AD_DLL_Phoibos_ListDeviceModes.vi"("dll path in"=w1465, "dev_type"=w1462, "pHandle"=w1463, "error in"=w1464) -> ("dll path out"=w1459:path, "error out"=w1458:errorcluster)  [unwired: 1 in, 2 out]
          }
          frame #2 {
            n743 = local write "phoib_con?"(TRUE ("phoib_con?")) -> ()
          }
        }
      }
    }
    "phoib_error" <- w1337
  }
